vi "4.0.3_Airwatts_Finetune.vi"(6 "Data in":T1, 8 "error in (no error)":errorcluster, 9 "AllControls In":T2, 10 "?":T3, 11 "Message Queue out":T4) -> (0 "error out":errorcluster, 1 "Flow":string, 2 "Data":T3, 3 "Message Queue Out":T4, 4 "Data out":T1)   [LabVIEW 2017]
uses:
  Depends/AMC/subVIs/TypeDefs/amc_Message Queue.ctl
  Depends/AMC/subVIs/TypeDefs/amc_Message.ctl
  Depends/Tools/Keyed Array/Tools_KeyedArray KeyedArray.ctl
  Ctrls/Data.ctl
  Ctrls/AllControls.ctl
  Ctrls/CSV_Data.ctl
  DIPC 692 Daemon API/typdef/get_parameter.ctl
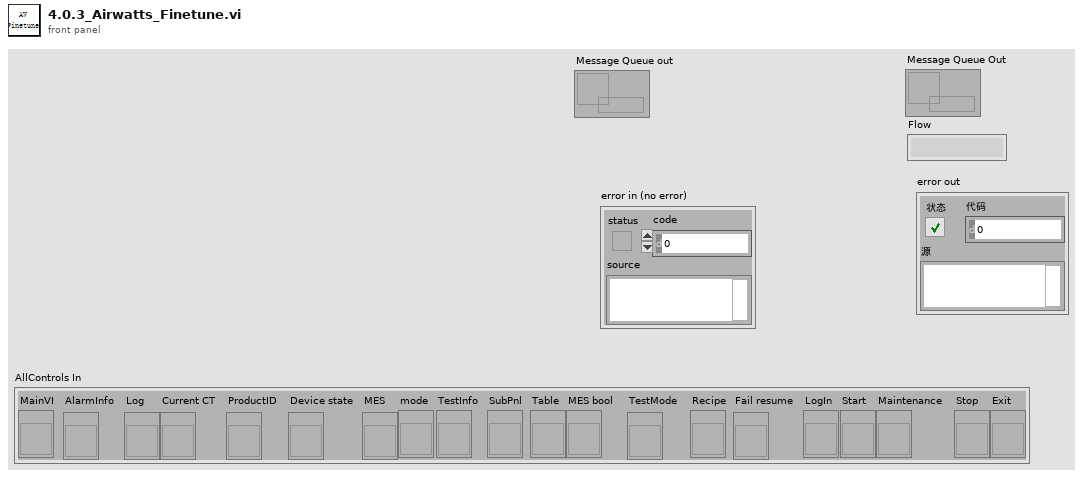
[diagram p1: front panel]
types:
  T1 = typedef "CSV_Data.ctl" = cluster{"Initialisation":cluster{"LMT - Connect UUT (con COM)":string, "LMT - Software Version (rrel)":string, "LMT - Write SKU file (wskuc)":string, "LMT - SKU file name":string, "Connect UUT DDM":string, "Read DDM EOL Timestamp - Mode":string, "Read DDM EOL Timestamp - Timestamp":string, "Read DDM EOL Timestamp - Rig ID":string, "Read DDM EOL Timestamp - Passmark ID":string, "Read DDM EOL Timestamp - Passmark Rev":string, "Software Version before flashing":string, "Read Hardware Serial":string, "UUT DDM SN":string, "Compare DDM SN with MES SN":string, "Backup PCBA Calibration EEPROM Response - CAL":string, "Flash Firmware Version":string, "Check SW Version":string, "Read DDM SW Version after flashing":string, "Set SKU Config":string, "Ready Status":string, "Set Device Mode to EOL":string, "DDM Parameter - Voltage":string, "DDM Parameter - Current":string, "DDM Parameter - Power":string, "DDM Parameter - Speed":string, "DDM Parameter - Pressure":string, "Tester Parameter - Voltage":string, "Tester Parameter - Current":string, "Tester Parameter - Power":string, "Tester Parameter - Ambient Pressure":string, "Tester Parameter - Ambient Temperature":string, "Calculated Parameter - DDM Pressure Corrected":string, "Calculated Parameter - DDM Real Power":string, "Calculated Parameter - Delta V":string}, "BEMF_Calibration":cluster{"Calibration Result - eol_cold_bemf_temp":string, "DDM Ambient Temp":string, "Restriction Plate Diameter":string, "Calibration Result - eol_bemf_mp_cold_coef_a":string, "Calibration Result - eol_bemf_mp_cold_coef_b":string, "Calibration Result - eol_bemf_mp_cold_coef_c":string, "Calibration Result - eol_bemf_lsi_cold_ref_coeffs":string, "Get - Calibration Result - eol_bemf_lsi_speed":string, "Get - Calibration Result - eol_bemf_lsi_integral_0":string, "Calibration Result - eol_bemf_lsi_integral_1":string, "Get - Calibration Result - eol_bemf_lsi_integral_2":string, "Get - Calibration Result - eol_cold_bemf":string, "Get - Calibration Result - eol_cold_bemf_fisf":string, "Finalise Calibration":string, "Compare -Calibration Result - eol_cold_bemf":string, "Compare -Calibration Result - eol_cold_bemf_fisf":string}, "ECO":cluster{"Reset Power Tune":string, "Reset BEMF FISF Calibration":string, "Restriction Plate Diameter":string, "ECO - Stabilisation Time":string, "ECO - DDM Parameter - Voltage":string, "ECO - DDM Parameter - Current":string, "ECO - DDM Parameter - Power":string, "ECO - DDM Parameter - Measured Power":string, "ECO - DDM Parameter - Speed":string, "ECO - DDM Parameter - Pressure":string, "ECO - Tester Parameter - Voltage":string, "ECO - Tester Parameter - Current":string, "ECO - Tester Parameter - Power":string, "ECO - Tester Parameter - Ambient Pressure":string, "ECO - Tester Parameter - Ambient Temperature":string, "ECO - Tester Parameter - Ambient Humidity":string, "ECO - Calculated Parameter - DDM Pressure Corrected":string, "ECO - Calculated Parameter - DDM Real Power":string, "ECO - Calculated Parameter - Delta V":string, "ECO - Calculated Parameter - Flowrate":string, "ECO - Calculated Parameter - Airwatt":string, "ECO - Formula":string, "PT ECO - Power Tune Mode Status":string}, "BOOST":cluster{"Restriction Plate Diameter":string, "BOOST - Stabilisation Time":string, "BOOST - DDM Parameter - Voltage":string, "BOOST - DDM Parameter - Current":string, "BOOST - DDM Parameter - Power":string, "BOOST - DDM Parameter - Measured Power":string, "BOOST - DDM Parameter - Speed":string, "BOOST - DDM Parameter - Pressure":string, "BOOST - Tester Parameter - Voltage":string, "BOOST - Tester Parameter - Current":string, "BOOST - Tester Parameter - Power":string, "BOOST - Tester Parameter - Ambient Pressure":string, "BOOST - Tester Parameter - Ambient Temperature":string, "BOOST - Tester Parameter - Ambient Humidity":string, "BOOST - Calculated Parameter - DDM Pressure Corrected":string, "BOOST - Calculated Parameter - DDM Real Power":string, "BOOST - Calculated Parameter - Delta V":string, "BOOST - Calculated Parameter - Flowrate":string, "BOOST - Calculated Parameter - Airwatt":string, "BOOST - Get AM Presence":string, "Air Muscle Turn Off Status":string, "BOOST - Air Muscle Calculated Parameter - Airwatt B":string, "BOOST - Air Muscle Calculate Airwatt Delta":string, "PT BOOST - Power Tune Mode Status":string, "Finalise Calibration":string, "ECO - Get AW Calibration value":string, "BOOST - Get AW Calibration value":string}, "MAX":cluster{"Restriction Plate Diameter":string, "MAX - Stabilisation Time":string, "Get Average Delta Tmag (LSIdelta_FISFdelta_LSItmag_FISFtmag_IIRtmag)":string, "Get Average Delta Tmag FISF":string, "MAX - DDM Parameter - Voltage":string, "MAX - DDM Parameter - Current":string, "MAX - DDM Parameter - Power":string, "MAX - DDM Parameter - Measured Power":string, "MAX - DDM Parameter - Speed":string, "MAX - DDM Parameter - Pressure":string, "MAX - Tester Parameter - Voltage":string, "MAX - Tester Parameter - Current":string, "MAX - Tester Parameter - Power":string, "MAX - Tester Parameter - Ambient Pressure":string, "MAX - Tester Parameter - Ambient Temperature":string, "MAX - Tester Parameter - Ambient Humidity":string, "MAX - Calculated Parameter - DDM Pressure Corrected":string, "MAX - Calculated Parameter - DDM Real Power":string, "MAX - Calculated Parameter - Delta V":string, "MAX - Calculated Parameter - Flowrate":string, "MAX - Calculated Parameter - Airwatt":string, "MAX_FISF_Check_Average_Delta_Tmag":string, "MAX - FISF - BEMF Finetune Result":string, "MAX tune - Delta P1":string, "MAX tune - Calculated Parameter - Airwatt":string, "Calculate Delta Airwatts - MAX finetune - Delta P2":string, "MAX finetune - DDM Parameter - Voltage":string, "MAX finetune - DDM Parameter - Current":string, "MAX finetune - DDM Parameter - Power":string, "MAX finetune - DDM Parameter - Measured Power":string, "MAX finetune - DDM Parameter - Speed":string, "MAX finetune - DDM Parameter - Pressure":string, "MAX finetune - Tester Parameter - Voltage":string, "MAX finetune - Tester Parameter - Current":string, "MAX finetune - Tester Parameter - Power":string, "MAX finetune - Tester Parameter - Ambient Pressure":string, "MAX finetune - Tester Parameter - Ambient Temperature":string, "MAX finetune - Tester Parameter - Ambient Humidity":string, "MAX finetune - Calculated Parameter - DDM Pressure Corrected":string, "MAX finetune - Calculated Parameter - DDM Real Power":string, "MAX finetune - Calculated Parameter - Delta V":string, "MAX finetune - Calculated Parameter - Flowrate":string, "MAX finetune - Calculated Parameter - Airwatt":string, "Check Derate Result":string, "Delta Tmag FISF":string, "Get Hot BEMF Result":string, "Calculate delta Pressure":string, "Finalise Calibration":string, "Calculate & Check Delta BEMF":string, "Delta P Airwatts Value":string}, "LL":cluster{"DDM Ambient Temp":string, "Restriction Plate Diameter":string, "LL - DDM Parameter - Voltage":string, "LL - DDM Parameter - Current":string, "LL - DDM Parameter - Power":string, "LL - DDM Parameter - Measured Power":string, "LL - DDM Parameter - Speed":string, "LL - DDM Parameter - Pressure":string, "LL - Tester Parameter - Voltage":string, "LL - Tester Parameter - Current":string, "LL - Tester Parameter - Power":string, "LL - DDM Real Power":string, "LL - Calibrate Task Detect LL":string}, "HL":cluster{"HL - DDM Parameter - Voltage":string, "HL - DDM Parameter - Current":string, "HL - DDM Parameter - Power":string, "HL - DDM Parameter - Measured Power":string, "HL - DDM Parameter - Speed":string, "HL - DDM Parameter - Pressure":string, "HL - Tester Parameter - Voltage":string, "HL - Tester Parameter - Current":string, "HL - Tester Parameter - Power":string, "HL - DDM Real Power":string, "HL - Calibrate Task Detect HL":string}, "LH":cluster{"Restriction Plate Diameter":string, "LH - DDM Parameter - Voltage":string, "LH - DDM Parameter - Current":string, "LH - DDM Parameter - Power":string, "LH - DDM Parameter - Measured Power":string, "LH - DDM Parameter - Speed":string, "LH - DDM Parameter - Pressure":string, "LH - Tester Parameter - Voltage":string, "LH - Tester Parameter - Current":string, "LH - Tester Parameter - Power":string, "LH - DDM Real Power":string, "LH - Calibrate Task Detect LH":string}, "HH":cluster{"HH - DDM Parameter - Voltage":string, "HH - DDM Parameter - Current":string, "HH - DDM Parameter - Power":string, "HH - DDM Parameter - Measured Power":string, "HH - DDM Parameter - Speed":string, "HH - DDM Parameter - Pressure":string, "HH - Tester Parameter - Voltage":string, "HH - Tester Parameter - Current":string, "HH - Tester Parameter - Power":string, "HH - DDM Real Power":string, "HH - Calibrate Task Detect HH":string}, "Inlet Blockage Calibration":cluster{"Inlet Blockage Calibration - DDM Parameter - Voltage":string, "Inlet Blockage Calibration - DDM Parameter - Current":string, "Inlet Blockage Calibration - DDM Parameter - Power":string, "Inlet Blockage Calibration - DDM Parameter - Measured Power":string, "Inlet Blockage Calibration - DDM Parameter - Speed":string, "Inlet Blockage Calibration - DDM Parameter - Pressure":string, "Inlet Blockage Calibration - Tester Parameter - Voltage":string, "Inlet Blockage Calibration - Tester Parameter - Current":string, "Inlet Blockage Calibration - Tester Parameter - Power":string, "Inlet Blockage Calibration - DDM Real Power":string, "Calibration Inlet Blockage_E":string, "Finalise Calibration":string, "Get Task Detect LL":string, "Get Task Detect HL":string, "Get Task Detect LH":string, "Get Task Detect HH":string, "Calibration Inlet Blockage":string, "Calibration eol cold bemf temp":string}, "GOOD":cluster{"GOOD UNIT - Clear EEPROM Error Log":string, "GOOD UNIT - Write Product Timestamp - Mode":string, "GOOD UNIT - Write Product Timestamp - Timestamp":string, "GOOD UNIT - Write Product Timestamp - Rig ID":string, "GOOD UNIT - Write Product Timestamp - Passmark ID":string, "GOOD UNIT - Write Product Timestamp - Passmark Rev":string, "GOOD UNIT - Set Device Mode to PROD":string, "GOOD UNIT - Backup PCBA Calibration EEPROM Response":string, "GOOD UNIT - Check Security Bit":string, "GOOD UNIT - Set Calibration Lock":string, "GOOD UNIT - Get_Calibration_Lock":string, "GOOD UNIT - Disconnect UUT":string}, "NG":cluster{"NG UNIT - Read NVM Error":string, "NG UNIT - Set Device Mode to FCT":string, "NG UNIT - Backup PCBA Calibration EEPROM Response - CAL":string, "NG UNIT - Backup PCBA Calibration EEPROM Response - ERROR":string, "NG UNIT - Backup PCBA Calibration EEPROM Response - USAGE":string, "NG UNIT - Disconnect UUT":string}, "SN":string, "Table":string[][], "Count":cluster{"Total":i32, "OK":i32, "NG":i32, "Yield":dbl}, "Start Time":timestamp, "daemon reference":refnum<k5>, "CT":dbl, "Config":string[][], "OK/NG":bool, "Station ID":string, "MES DDM SN":string, "MES PCBA SN":string, "Retest":string, "UID":string, "Initialisation_Status":cluster{"LMT - Connect UUT (con COM)":string, "LMT - Software Version (rrel)":string, "LMT - Write SKU file (wskuc)":string, "LMT - SKU file name":string, "Connect UUT DDM":string, "Read DDM EOL Timestamp - Mode":string, "Read DDM EOL Timestamp - Timestamp":string, "Read DDM EOL Timestamp - Rig ID":string, "Read DDM EOL Timestamp - Passmark ID":string, "Read DDM EOL Timestamp - Passmark Rev":string, "Software Version before flashing":string, "Read Hardware Serial":string, "UUT DDM SN":string, "Compare DDM SN with MES SN":string, "Backup PCBA Calibration EEPROM Response - CAL":string, "Flash Firmware Version":string, "Check SW Version":string, "Read DDM SW Version after flashing":string, "Set SKU Config":string, "Ready Status":string, "Set Device Mode to EOL":string, "DDM Parameter - Voltage":string, "DDM Parameter - Current":string, "DDM Parameter - Power":string, "DDM Parameter - Speed":string, "DDM Parameter - Pressure":string, "Tester Parameter - Voltage":string, "Tester Parameter - Current":string, "Tester Parameter - Power":string, "Tester Parameter - Ambient Pressure":string, "Tester Parameter - Ambient Temperature":string, "Calculated Parameter - DDM Pressure Corrected":string, "Calculated Parameter - DDM Real Power":string, "Calculated Parameter - Delta V":string}, "BEMF_Calibration_Status":cluster{"Calibration Result - eol_cold_bemf_temp":string, "DDM Ambient Temp":string, "Restriction Plate Diameter":string, "Calibration Result - eol_bemf_mp_cold_coef_a":string, "Calibration Result - eol_bemf_mp_cold_coef_b":string, "Calibration Result - eol_bemf_mp_cold_coef_c":string, "Calibration Result - eol_bemf_lsi_cold_ref_coeffs":string, "Get - Calibration Result - eol_bemf_lsi_speed":string, "Get - Calibration Result - eol_bemf_lsi_integral_0":string, "Calibration Result - eol_bemf_lsi_integral_1":string, "Get - Calibration Result - eol_bemf_lsi_integral_2":string, "Get - Calibration Result - eol_cold_bemf":string, "Get - Calibration Result - eol_cold_bemf_fisf":string, "Finalise Calibration":string, "Compare -Calibration Result - eol_cold_bemf":string, "Compare -Calibration Result - eol_cold_bemf_fisf":string}, "ECO_Status":cluster{"Reset Power Tune":string, "Reset BEMF FISF Calibration":string, "Restriction Plate Diameter":string, "ECO - Stabilisation Time":string, "ECO - DDM Parameter - Voltage":string, "ECO - DDM Parameter - Current":string, "ECO - DDM Parameter - Power":string, "ECO - DDM Parameter - Measured Power":string, "ECO - DDM Parameter - Speed":string, "ECO - DDM Parameter - Pressure":string, "ECO - Tester Parameter - Voltage":string, "ECO - Tester Parameter - Current":string, "ECO - Tester Parameter - Power":string, "ECO - Tester Parameter - Ambient Pressure":string, "ECO - Tester Parameter - Ambient Temperature":string, "ECO - Tester Parameter - Ambient Humidity":string, "ECO - Calculated Parameter - DDM Pressure Corrected":string, "ECO - Calculated Parameter - DDM Real Power":string, "ECO - Calculated Parameter - Delta V":string, "ECO - Calculated Parameter - Flowrate":string, "ECO - Calculated Parameter - Airwatt":string, "ECO - Formula":string, "PT ECO - Power Tune Mode Status":string}, "BOOST_Status":cluster{"Restriction Plate Diameter":string, "BOOST - Stabilisation Time":string, "BOOST - DDM Parameter - Voltage":string, "BOOST - DDM Parameter - Current":string, "BOOST - DDM Parameter - Power":string, "BOOST - DDM Parameter - Measured Power":string, "BOOST - DDM Parameter - Speed":string, "BOOST - DDM Parameter - Pressure":string, "BOOST - Tester Parameter - Voltage":string, "BOOST - Tester Parameter - Current":string, "BOOST - Tester Parameter - Power":string, "BOOST - Tester Parameter - Ambient Pressure":string, "BOOST - Tester Parameter - Ambient Temperature":string, "BOOST - Tester Parameter - Ambient Humidity":string, "BOOST - Calculated Parameter - DDM Pressure Corrected":string, "BOOST - Calculated Parameter - DDM Real Power":string, "BOOST - Calculated Parameter - Delta V":string, "BOOST - Calculated Parameter - Flowrate":string, "BOOST - Calculated Parameter - Airwatt":string, "BOOST - Get AM Presence":string, "Air Muscle Turn Off Status":string, "BOOST - Air Muscle Calculated Parameter - Airwatt B":string, "BOOST - Air Muscle Calculate Airwatt Delta":string, "PT BOOST - Power Tune Mode Status":string, "Finalise Calibration":string, "ECO - Get AW Calibration value":string, "BOOST - Get AW Calibration value":string}, "MAX_Status":cluster{"Restriction Plate Diameter":string, "MAX - Stabilisation Time":string, "Get Average Delta Tmag (LSIdelta_FISFdelta_LSItmag_FISFtmag_IIRtmag)":string, "Get Average Delta Tmag FISF":string, "MAX - DDM Parameter - Voltage":string, "MAX - DDM Parameter - Current":string, "MAX - DDM Parameter - Power":string, "MAX - DDM Parameter - Measured Power":string, "MAX - DDM Parameter - Speed":string, "MAX - DDM Parameter - Pressure":string, "MAX - Tester Parameter - Voltage":string, "MAX - Tester Parameter - Current":string, "MAX - Tester Parameter - Power":string, "MAX - Tester Parameter - Ambient Pressure":string, "MAX - Tester Parameter - Ambient Temperature":string, "MAX - Tester Parameter - Ambient Humidity":string, "MAX - Calculated Parameter - DDM Pressure Corrected":string, "MAX - Calculated Parameter - DDM Real Power":string, "MAX - Calculated Parameter - Delta V":string, "MAX - Calculated Parameter - Flowrate":string, "MAX - Calculated Parameter - Airwatt":string, "MAX_FISF_Check_Average_Delta_Tmag":string, "MAX - FISF - BEMF Finetune Result":string, "MAX tune - Delta P1":string, "MAX tune - Calculated Parameter - Airwatt":string, "Calculate Delta Airwatts - MAX finetune - Delta P2":string, "MAX finetune - DDM Parameter - Voltage":string, "MAX finetune - DDM Parameter - Current":string, "MAX finetune - DDM Parameter - Power":string, "MAX finetune - DDM Parameter - Measured Power":string, "MAX finetune - DDM Parameter - Speed":string, "MAX finetune - DDM Parameter - Pressure":string, "MAX finetune - Tester Parameter - Voltage":string, "MAX finetune - Tester Parameter - Current":string, "MAX finetune - Tester Parameter - Power":string, "MAX finetune - Tester Parameter - Ambient Pressure":string, "MAX finetune - Tester Parameter - Ambient Temperature":string, "MAX finetune - Tester Parameter - Ambient Humidity":string, "MAX finetune - Calculated Parameter - DDM Pressure Corrected":string, "MAX finetune - Calculated Parameter - DDM Real Power":string, "MAX finetune - Calculated Parameter - Delta V":string, "MAX finetune - Calculated Parameter - Flowrate":string, "MAX finetune - Calculated Parameter - Airwatt":string, "Check Derate Result":string, "Delta Tmag FISF":string, "Get Hot BEMF Result":string, "Calculate delta Pressure":string, "Finalise Calibration":string, "Calculate & Check Delta BEMF":string, "Delta P Airwatts Value":string}, "LL_Status":cluster{"DDM Ambient Temp":string, "Restriction Plate Diameter":string, "LL - DDM Parameter - Voltage":string, "LL - DDM Parameter - Current":string, "LL - DDM Parameter - Power":string, "LL - DDM Parameter - Measured Power":string, "LL - DDM Parameter - Speed":string, "LL - DDM Parameter - Pressure":string, "LL - Tester Parameter - Voltage":string, "LL - Tester Parameter - Current":string, "LL - Tester Parameter - Power":string, "LL - DDM Real Power":string, "LL - Calibrate Task Detect LL":string}, "HL_Status":cluster{"HL - DDM Parameter - Voltage":string, "HL - DDM Parameter - Current":string, "HL - DDM Parameter - Power":string, "HL - DDM Parameter - Measured Power":string, "HL - DDM Parameter - Speed":string, "HL - DDM Parameter - Pressure":string, "HL - Tester Parameter - Voltage":string, "HL - Tester Parameter - Current":string, "HL - Tester Parameter - Power":string, "HL - DDM Real Power":string, "HL - Calibrate Task Detect HL":string}, "LH_Status":cluster{"Restriction Plate Diameter":string, "LH - DDM Parameter - Voltage":string, "LH - DDM Parameter - Current":string, "LH - DDM Parameter - Power":string, "LH - DDM Parameter - Measured Power":string, "LH - DDM Parameter - Speed":string, "LH - DDM Parameter - Pressure":string, "LH - Tester Parameter - Voltage":string, "LH - Tester Parameter - Current":string, "LH - Tester Parameter - Power":string, "LH - DDM Real Power":string, "LH - Calibrate Task Detect LH":string}, "HH_Status":cluster{"HH - DDM Parameter - Voltage":string, "HH - DDM Parameter - Current":string, "HH - DDM Parameter - Power":string, "HH - DDM Parameter - Measured Power":string, "HH - DDM Parameter - Speed":string, "HH - DDM Parameter - Pressure":string, "HH - Tester Parameter - Voltage":string, "HH - Tester Parameter - Current":string, "HH - Tester Parameter - Power":string, "HH - DDM Real Power":string, "HH - Calibrate Task Detect HH":string}, "Inlet Blockage Calibration_Status":cluster{"Inlet Blockage Calibration - DDM Parameter - Voltage":string, "Inlet Blockage Calibration - DDM Parameter - Current":string, "Inlet Blockage Calibration - DDM Parameter - Power":string, "Inlet Blockage Calibration - DDM Parameter - Measured Power":string, "Inlet Blockage Calibration - DDM Parameter - Speed":string, "Inlet Blockage Calibration - DDM Parameter - Pressure":string, "Inlet Blockage Calibration - Tester Parameter - Voltage":string, "Inlet Blockage Calibration - Tester Parameter - Current":string, "Inlet Blockage Calibration - Tester Parameter - Power":string, "Inlet Blockage Calibration - DDM Real Power":string, "Calibration Inlet Blockage_E":string, "Finalise Calibration":string, "Get Task Detect LL":string, "Get Task Detect HL":string, "Get Task Detect LH":string, "Get Task Detect HH":string, "Calibration Inlet Blockage":string, "Calibration eol cold bemf temp":string}, "GOOD_Status":cluster{"GOOD UNIT - Clear EEPROM Error Log":string, "GOOD UNIT - Write Product Timestamp - Mode":string, "GOOD UNIT - Write Product Timestamp - Timestamp":string, "GOOD UNIT - Write Product Timestamp - Rig ID":string, "GOOD UNIT - Write Product Timestamp - Passmark ID":string, "GOOD UNIT - Write Product Timestamp - Passmark Rev":string, "GOOD UNIT - Set Device Mode to PROD":string, "GOOD UNIT - Backup PCBA Calibration EEPROM Response":string, "GOOD UNIT - Check Security Bit":string, "GOOD UNIT - Set Calibration Lock":string, "GOOD UNIT - Get_Calibration_Lock":string, "GOOD UNIT - Disconnect UUT":string}, "NG_Status":cluster{"NG UNIT - Read NVM Error":string, "NG UNIT - Set Device Mode to FCT":string, "NG UNIT - Backup PCBA Calibration EEPROM Response - CAL":string, "NG UNIT - Backup PCBA Calibration EEPROM Response - ERROR":string, "NG UNIT - Backup PCBA Calibration EEPROM Response - USAGE":string, "NG UNIT - Disconnect UUT":string}, "SKU":string, "Plate_Diameter":string, "Alarm":string}
  T2 = typedef "AllControls.ctl" = cluster{"MainVI":refnum<vi>, "AlarmInfo":refnum<vi>, "Log":refnum<vi>, "Current CT":refnum<vi>, "ProductID":refnum<vi>, "Device state":refnum<vi>, "MES":refnum<vi>, "mode":refnum<vi>, "TestInfo":refnum<vi>, "SubPnl":refnum<vi>, "Table":refnum<vi>, "MES bool":refnum<vi>, "TestMode":refnum<vi>, "Recipe":refnum<vi>, "Fail resume":refnum<vi>, "LogIn":refnum<vi>, "Start":refnum<vi>, "Maintenance":refnum<vi>, "Stop":refnum<vi>, "Exit":refnum<vi>}
  T3 = typedef "Data.ctl" = cluster{"Initialisation":cluster{"DDM_Parameter":dbl[], "DDM_Parameter_status":bool[], "Get_Tester_Parameter":dbl[], "Get_Tester_Parameter_status":bool[], "Cal_Tester_Parameter":dbl[], "Cal_Tester_Parameter_status":bool[], "sw_version_before_status":bool, "sw_version_after_status":bool, "Set_SKU_Config_With_LMT_status":bool, "FCT_timestamp_status":bool, "LMT_Connect_to_UUT_status":bool}, "BEMF_Calibration":cluster{"Read_ambient_temperature":dbl, "Calibration_Vaule":dbl[], "Calibration_Vaule _B":dbl[], "Calibration_Vaule_status":bool[], "Calibration_Vaule_B_status":bool[]}, "ECO":cluster{"DDM_Parameter":dbl[], "DDM_Parameter_status":bool[], "Get_Tester_Parameter":dbl[], "Get_Tester_Parameter_status":bool[], "Cal_Tester_Parameter":dbl[], "Cal_Tester_Parameter_status":bool[], "DDM_Parameter_after_power_tune":dbl[], "Get_Tester_Parameter_after_power_tune":dbl[], "Cal_Tester_Parameter_after_power_tune":dbl[], "Cal_Tester_Parameter_after_power_tune_status":bool[], "Delta_P":dbl}, "BOOST":cluster{"DDM_Parameter":dbl[], "DDM_Parameter_status":bool[], "Get_Tester_Parameter":dbl[], "Get_Tester_Parameter_status":bool[], "Cal_Tester_Parameter":dbl[], "Cal_Tester_Parameter_status":bool[], "DDM_Parameter_after_power_tune":dbl[], "Get_Tester_Parameter_after_power_tune":dbl[], "Cal_Tester_Parameter_after_power_tune":dbl[], "Cal_Tester_Parameter_after_power_tune_status":bool[], "airwatts_am_off":dbl, "AW_Delta_(AM_on_and_off)":dbl, "AW_Delta_(AM_on_and_off)_Status":bool, "Delta_P":dbl}, "MAX":cluster{"Average_Tmag_Data":cluster{"LSI Delta in degC":dbl, "FISF Delta in degc":dbl, "LSI Tmag in degC":dbl, "Fisf Tmag in degC":dbl, "IIR Tmag in degC":dbl}, "DDM_Parameter":dbl[], "DDM_Parameter_status":bool[], "Get_Tester_Parameter":dbl[], "Get_Tester_Parameter_status":bool[], "Cal_Tester_Parameter":dbl[], "BEMF_Finetune":cluster{"eol_bemf_mp_cold_coef_c":dbl, "eol_cold_bemf_fisf_offset":dbl}, "AW_Tune":cluster{"delta_P1":dbl, "delta_P_Setting":dbl}, "DDM_Parameter_after_Airwatts_Tune":dbl[], "Get_Tester_Parameter_after_Airwatts_Tune":dbl[], "Cal_Tester_Parameter_after_Airwatts_Tune":dbl[], "DDM_Parameter_after_Airwatts_Finetune":dbl[], "Get_Tester_Parameter_after_Airwatts_Finetune":dbl[], "Cal_Tester_Parameter_after_Airwatts_Finetune":dbl[], "AW_Finetune":cluster{"delta_P2":dbl, "delta_P_Setting":dbl}, "Delta_Tmag_after_tune":cluster{"LSI Delta in degC":dbl, "FISF Delta in degc":dbl, "LSI Tmag in degC":dbl, "Fisf Tmag in degC":dbl, "IIR Tmag in degC":dbl}, "Hot Bemf in mV":dbl, "DDM_Pressure":dbl, "Delta_Pressure":dbl, " Cold Bemf in mV":dbl, " delta Bemf":dbl, " delta p":dbl, "Delta_Pressure_status":bool, " delta Bemf_status":bool, "LSI Delta in degC_status":bool, "FISF Delta in degc_status":bool, "Max_check_derate_status_status":bool, "Average_All_data":dbl[][], "Average_Tmag_Data_status":bool[], "Average_Tmag_Data_after_tune_status":bool[], "Cal_Tester_Parameter_status":bool[], "Cal_Tester_Parameter_status_after_Airwatts_Tune":bool[], "Cal_Tester_Parameter_status_after_Airwatts_FineTune":bool[]}, "Task_Detect_Calib":cluster{"LL":cluster{"DDM_Parameter":dbl[], "DDM_Parameter_status":bool[], "Get_Tester_Parameter":dbl[], "Get_Tester_Parameter_status":bool[], "Set_task_detect_A":dbl, "Set_task_detect_A_Status":bool}, "HL":cluster{"DDM_Parameter":dbl[], "DDM_Parameter_status":bool[], "Get_Tester_Parameter":dbl[], "Get_Tester_Parameter_status":bool[], "Set_task_detect_B":dbl, "Set_task_detect_B_Status":bool}, "LH":cluster{"DDM_Parameter":dbl[], "DDM_Parameter_status":bool[], "Get_Tester_Parameter":dbl[], "Get_Tester_Parameter_status":bool[], "Set_task_detect_C":dbl, "Set_task_detect_C_Status":bool}, "HH":cluster{"DDM_Parameter":dbl[], "DDM_Parameter_status":bool[], "Get_Tester_Parameter":dbl[], "Get_Tester_Parameter_status":bool[], "Set_task_detect_D":dbl, "Read_and_check_calibration_Status":bool[], "Set_task_detect_D_Status":bool}, "Get_eol_inlet_blockage_E":dbl, "Calib_vaule":cluster{"Get_task_detect_LL":dbl, "Get_task_detect_HL":dbl, "Get_task_detect_LH":dbl, "Get_task_detect_HH":dbl, "eol_inlet_blockage":dbl, "eol_code_bemf_temp":dbl}, "calibrated temp":dbl, "Inlet_Blockage_Calibration":cluster{"DDM_Parameter":dbl[], "DDM_Parameter_status":bool[], "Get_Tester_Parameter":dbl[], "Get_Tester_Parameter_status":bool[]}, "Get_eol_inlet_blockage_E_Status":bool}, "good":cluster{"Write_Product_TS":cluster{"TIMESTAMP":i64, "RIG_ID":i64, "PASSMARK_ID":i64, "PASSMARK_REV":i64}, "Read_Product_TS":cluster{"TIMESTAMP":i64, "RIG_ID":i64, "PASSMARK_ID":i64, "PASSMARK_REV":i64}, "Good_Check_Secuity_Bit_Stauts":bool}}
  T4 = typedef "amc_Message Queue.ctl" = refnum<queue>
  T5 = typedef "HD Config.ctl" = cluster{" PC":cluster{"PC Address":u8[], "PC Port":i32}, "FCO":cluster{"COM":refnum<visa-resource-name>, "Baudrate":u32}, "DC Power ":cluster{"COM":refnum<visa-resource-name>, "Baudrate":u32}, "PW3336":cluster{"COM":refnum<visa-resource-name>, "Baudrate":u32}, "Lefoo":cluster{"COM":refnum<visa-resource-name>, "Baudrate":u32}, "AI Model":cluster{"COM":refnum<visa-resource-name>, "Baudrate":u32}, "DIPC":cluster{"COM":refnum<visa-resource-name>}, "RFID":cluster{"IP Address":string, "Port":u16, "Retry":u16}, "Motor":cluster{"COM":refnum<visa-resource-name>, "Baudrate":u32}, "Fail_resume_mode":bool, "GRR":bool}
  T6 = cluster{"real_ddm_power_a_in_W":dbl, "real_ddm_power_b_in_W":dbl, "Target_AW":dbl, "AW extra":dbl, "latest_AW":dbl, "Correction_Factor":dbl, "P_extra in W":dbl, "delta_P index":dbl}
  T7 = typedef "get_parameter.ctl" = string
  T8 = cluster{"real_ddm_power_a_in_W":string, "real_ddm_power_b_in_W":string, "Target_AW":string, "AW extra":string, "latest_AW":string, "Correction_Factor":string, "P_extra in W":string, "delta_P index":string}
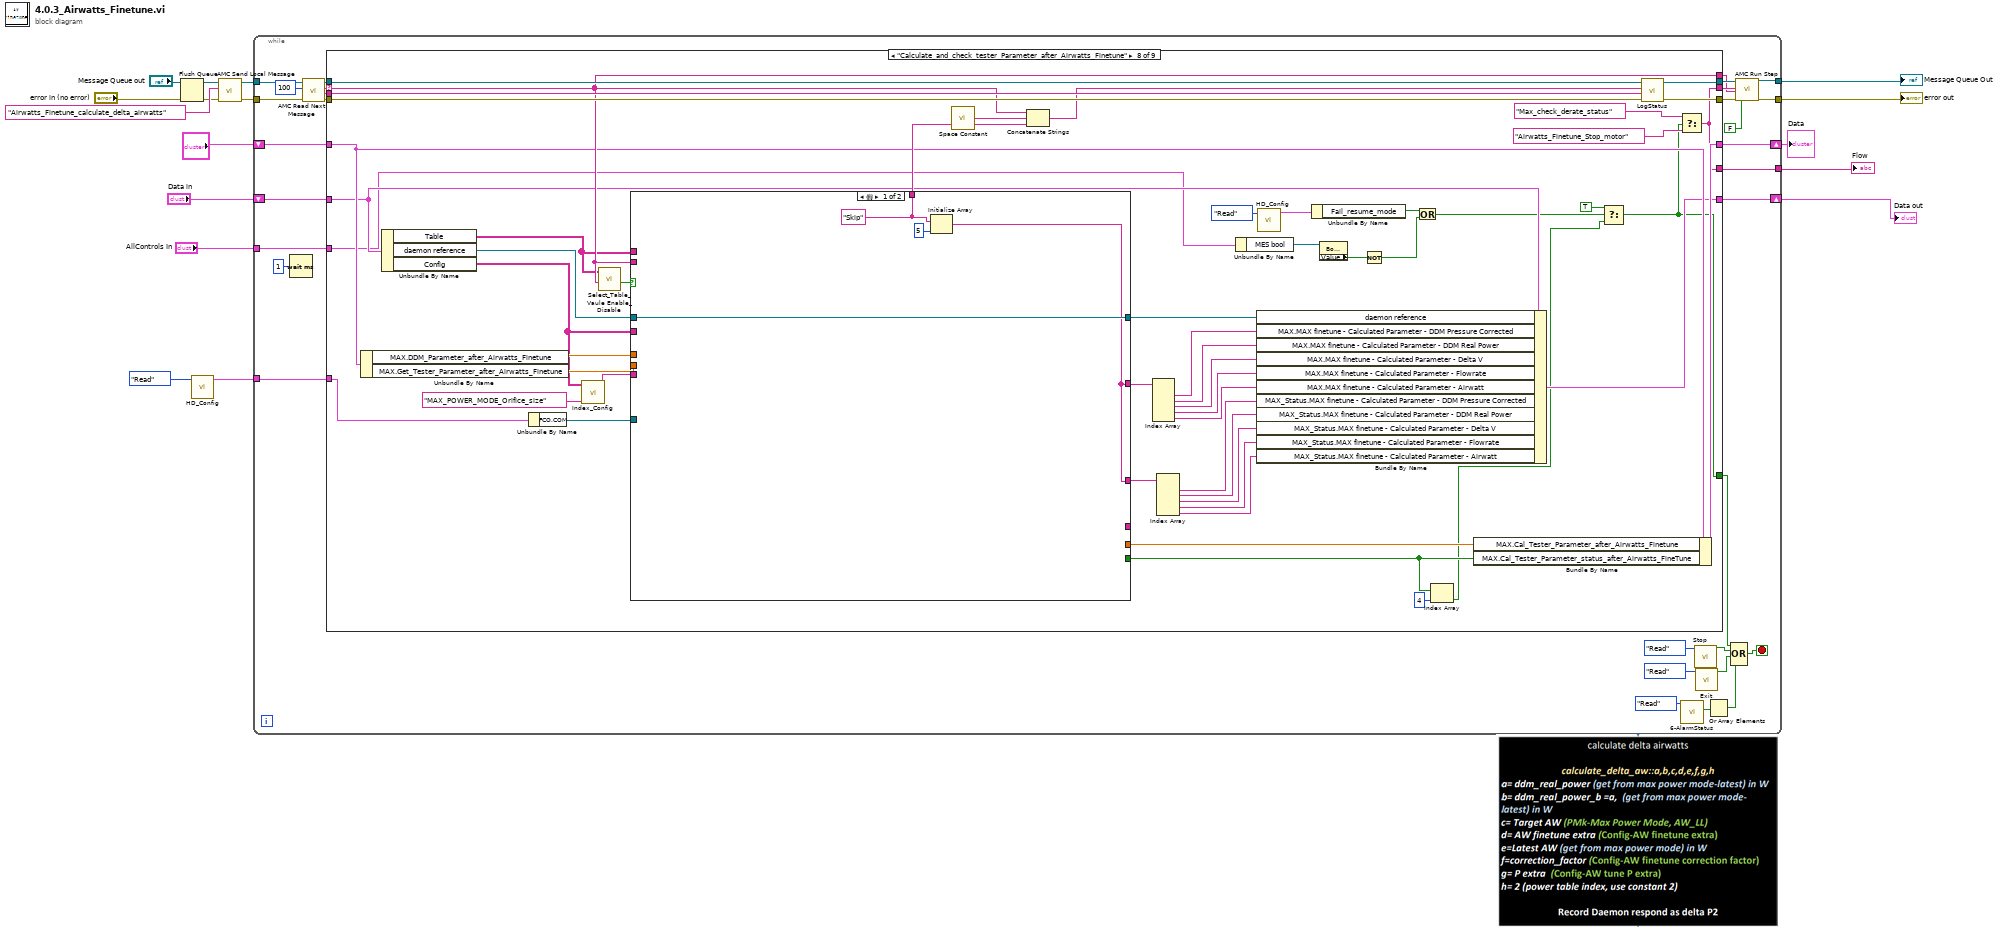
[diagram p0: block diagram]
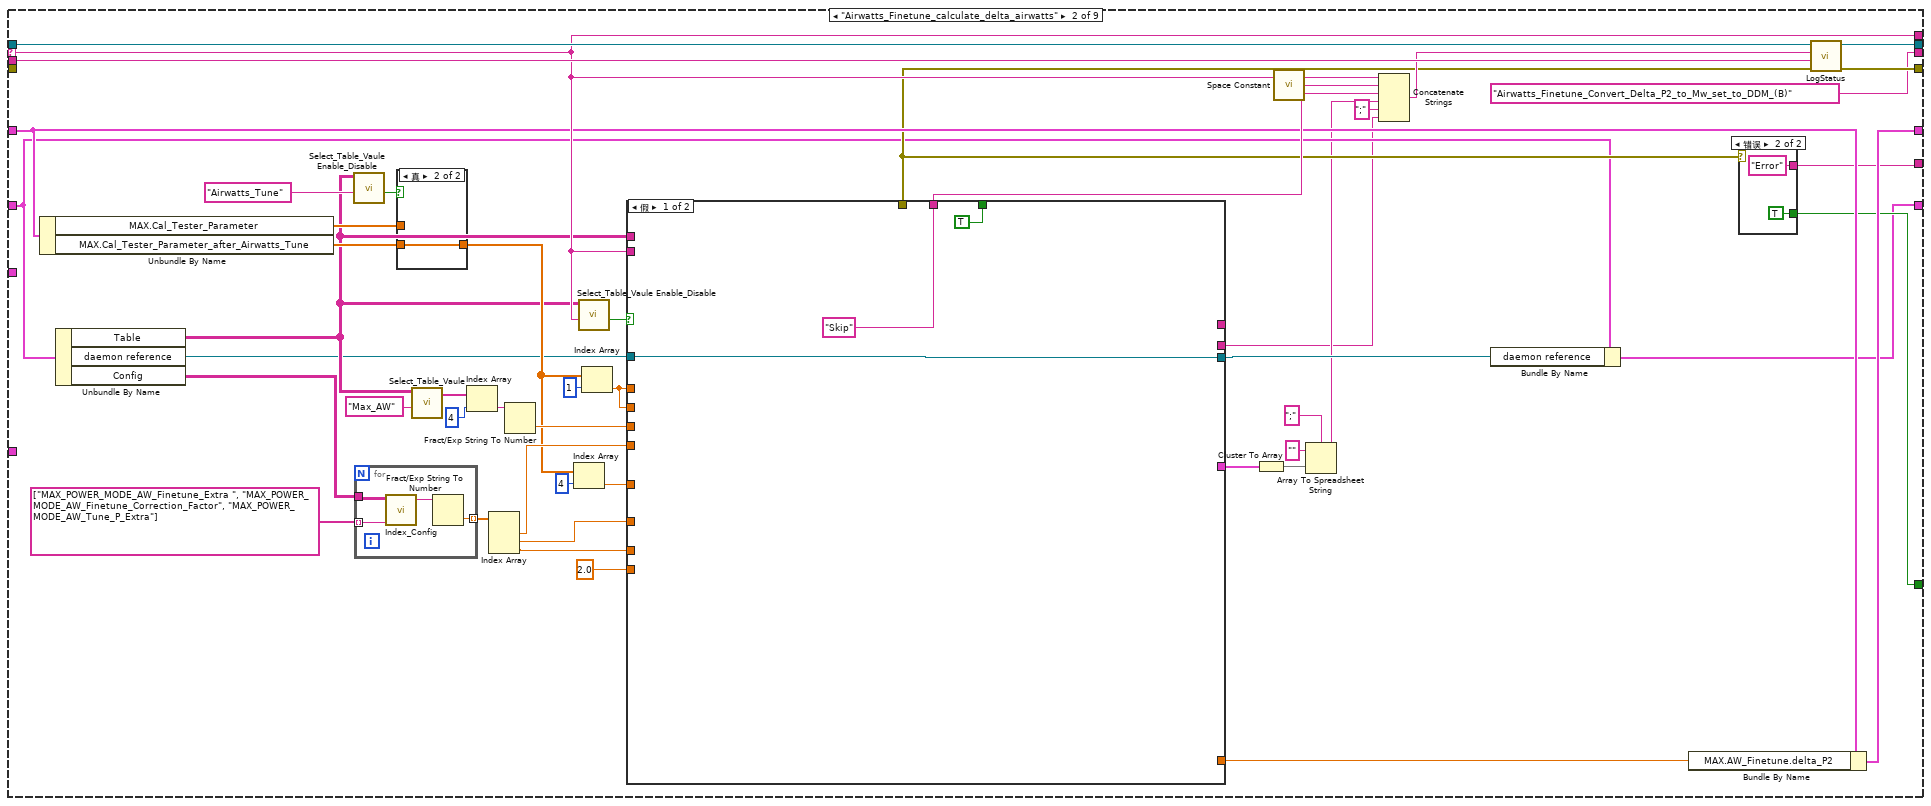
[diagram p3: hidden frame]
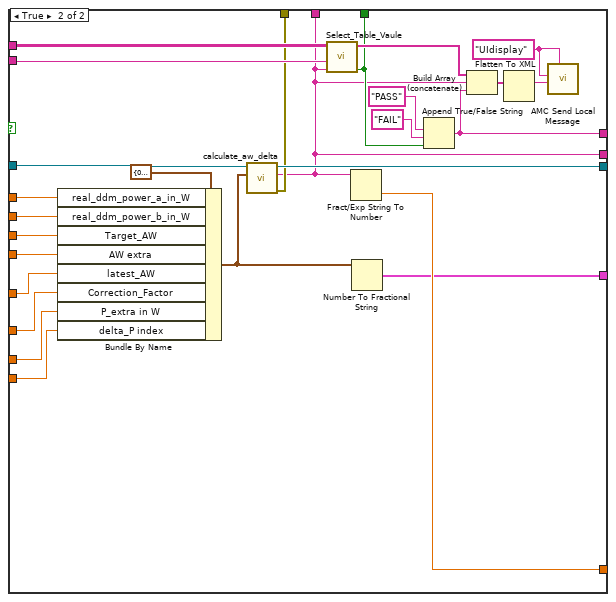
[diagram p6: hidden frame]
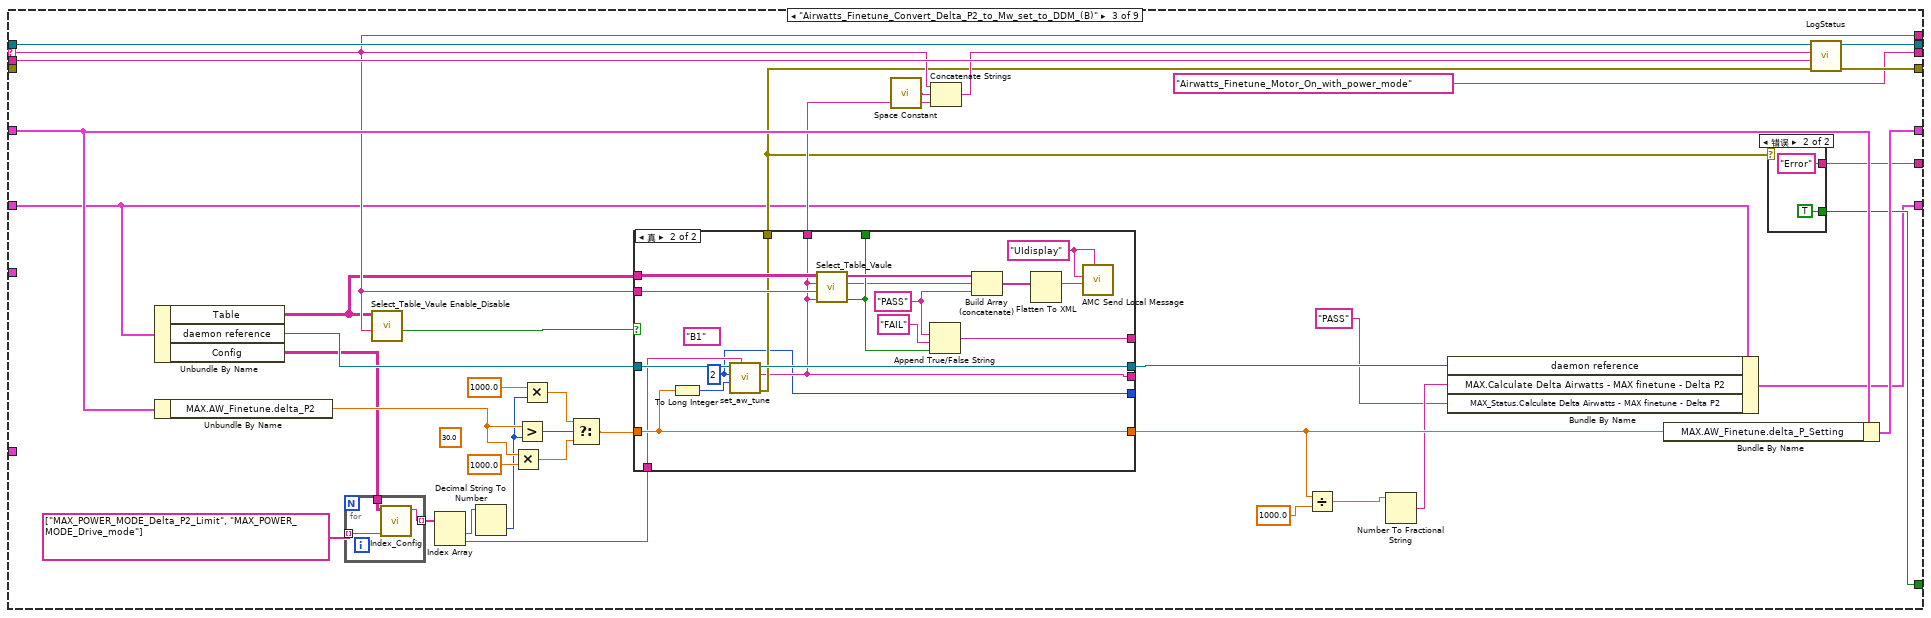
[diagram p7: hidden frame]
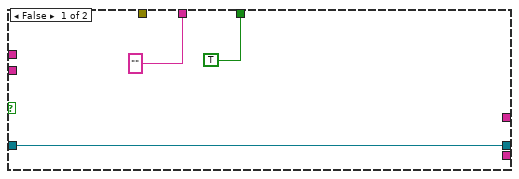
[diagram p9: hidden frame]
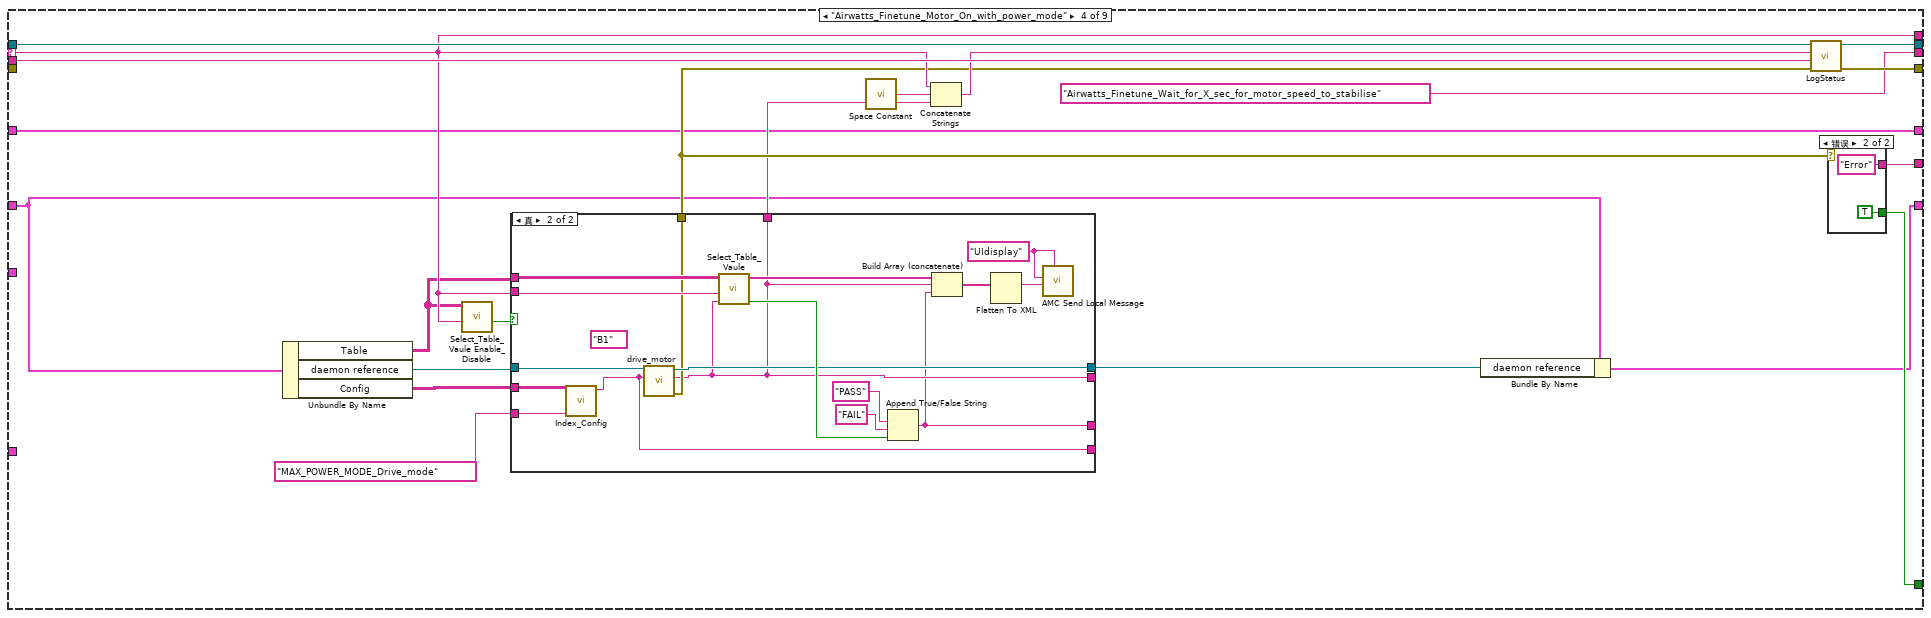
[diagram p10: hidden frame]
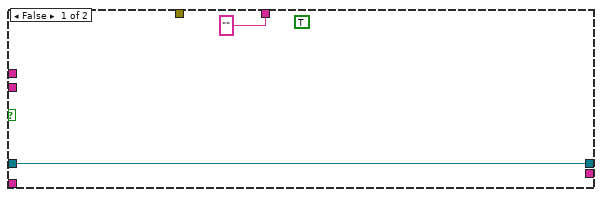
[diagram p12: hidden frame]
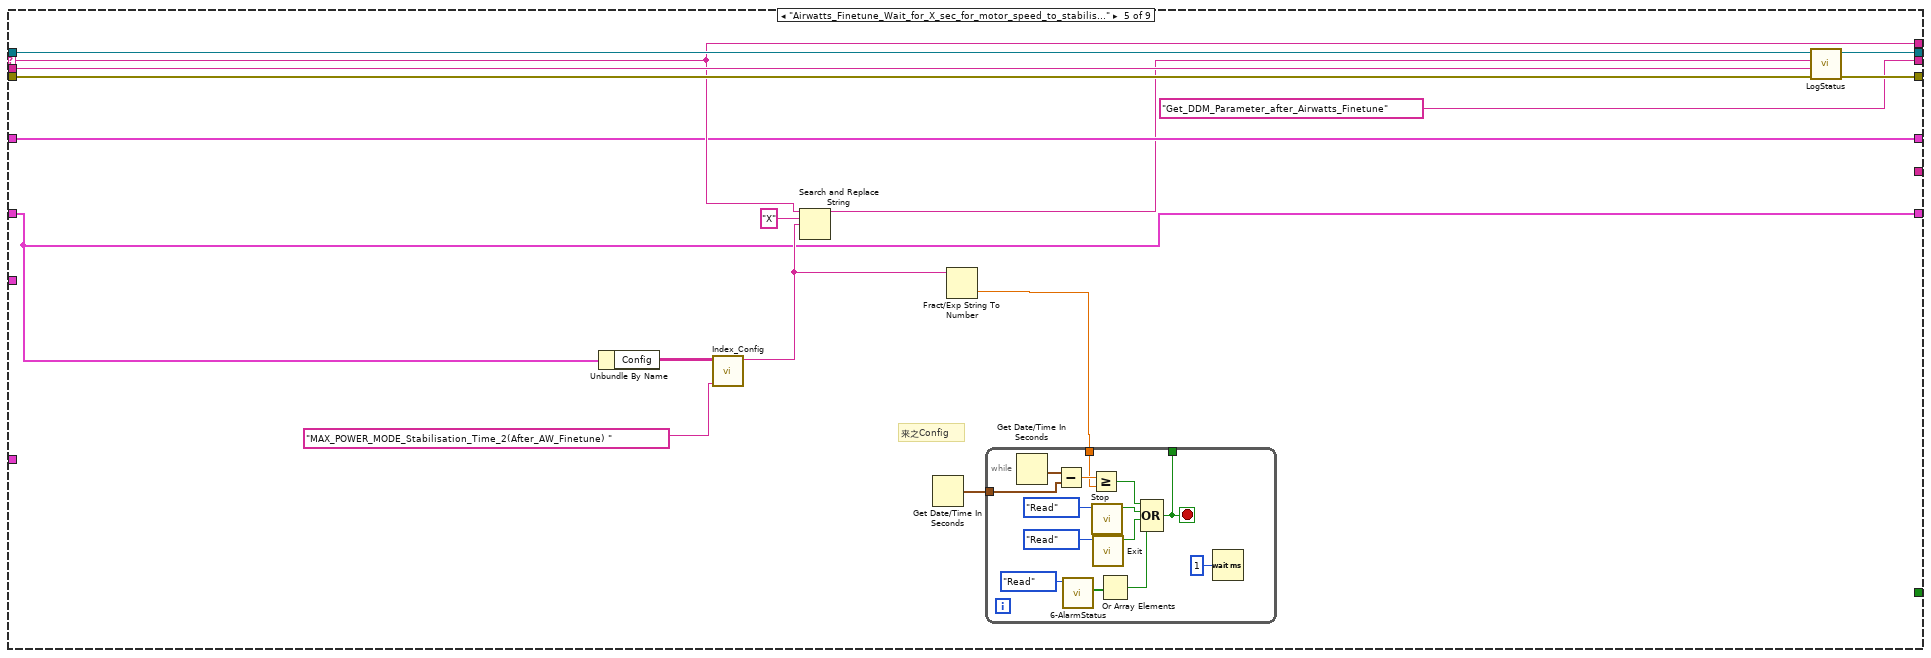
[diagram p13: hidden frame]
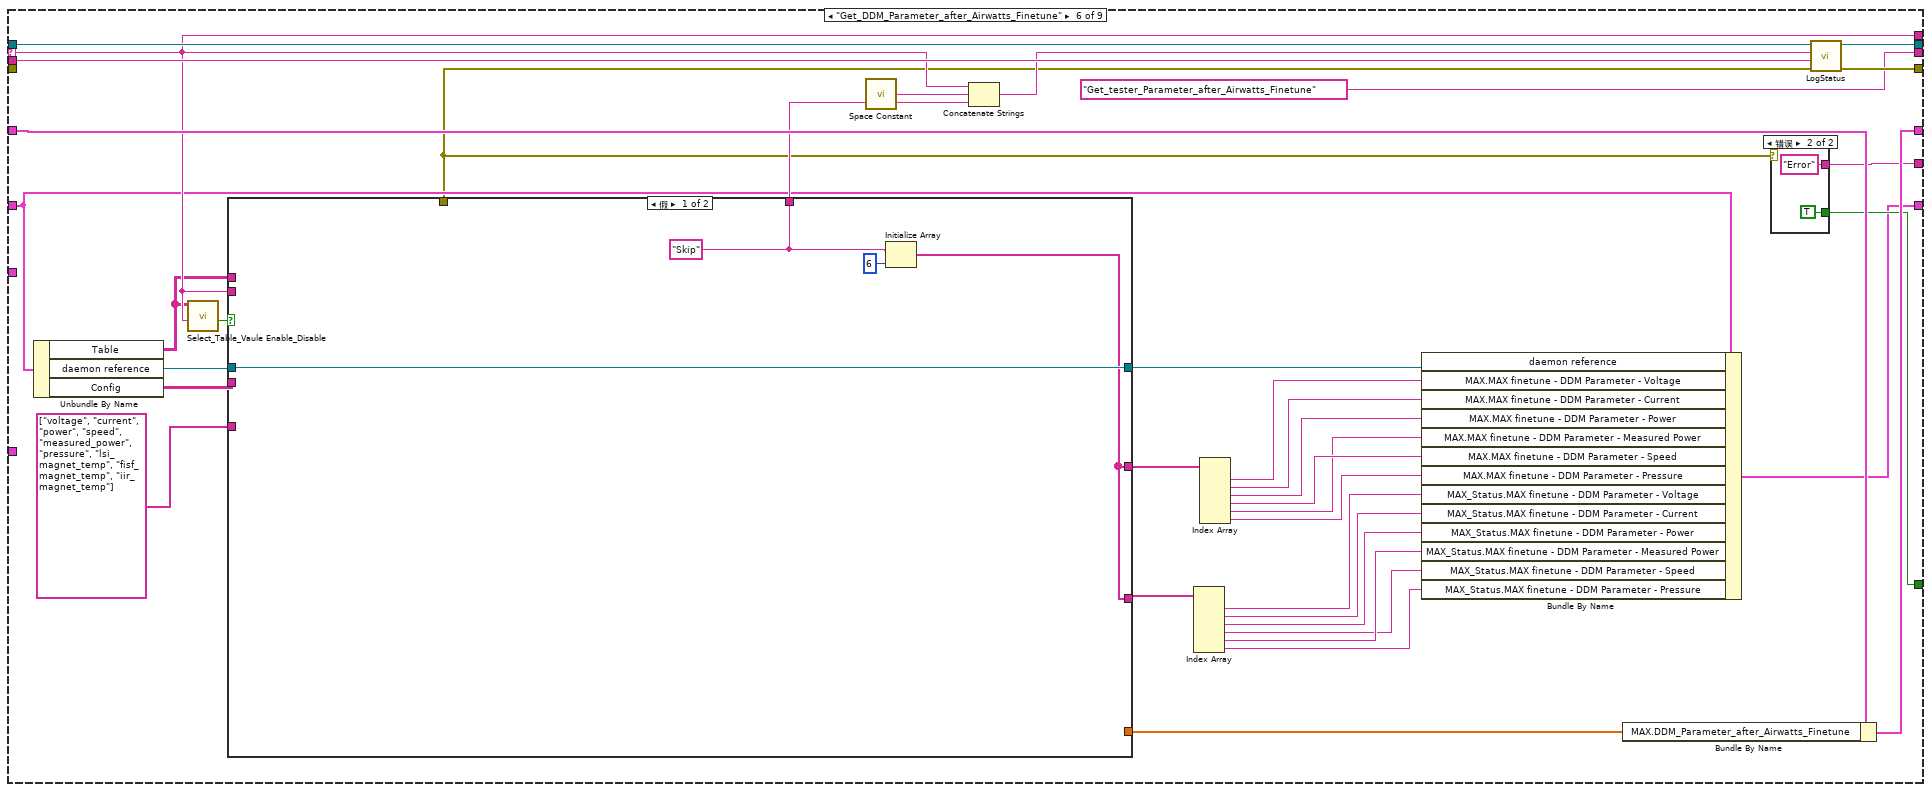
[diagram p14: hidden frame]
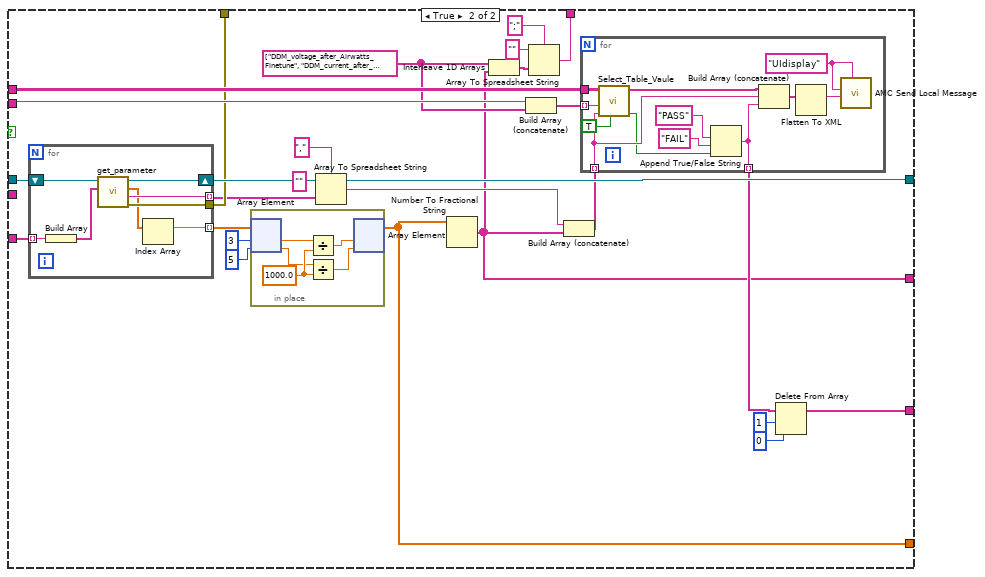
[diagram p16: hidden frame]
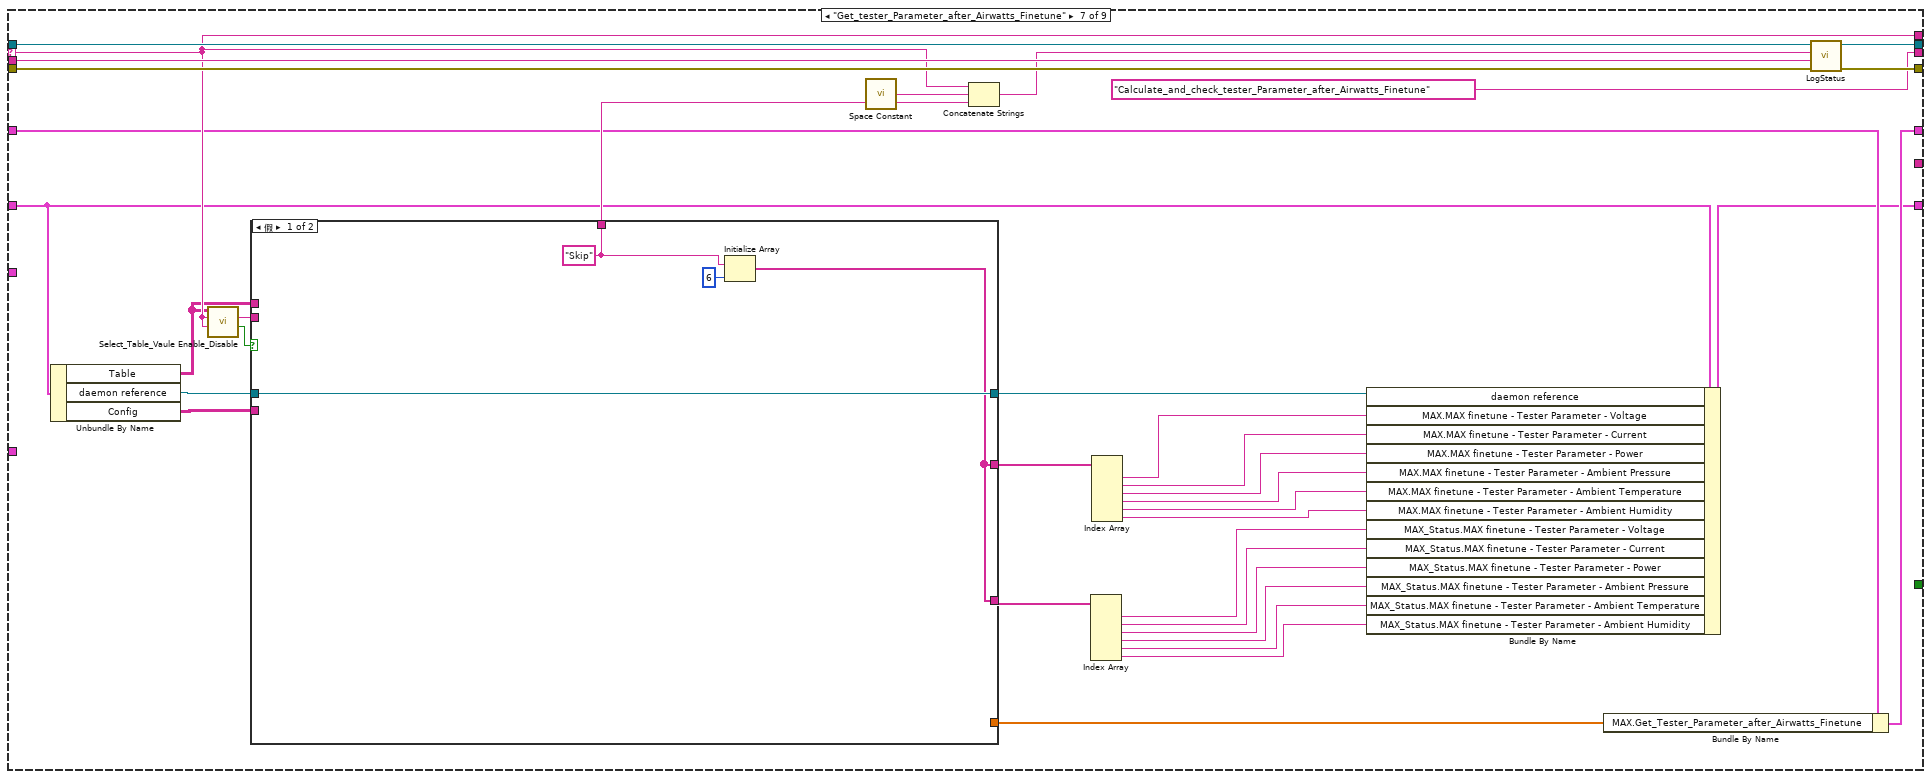
[diagram p17: hidden frame]
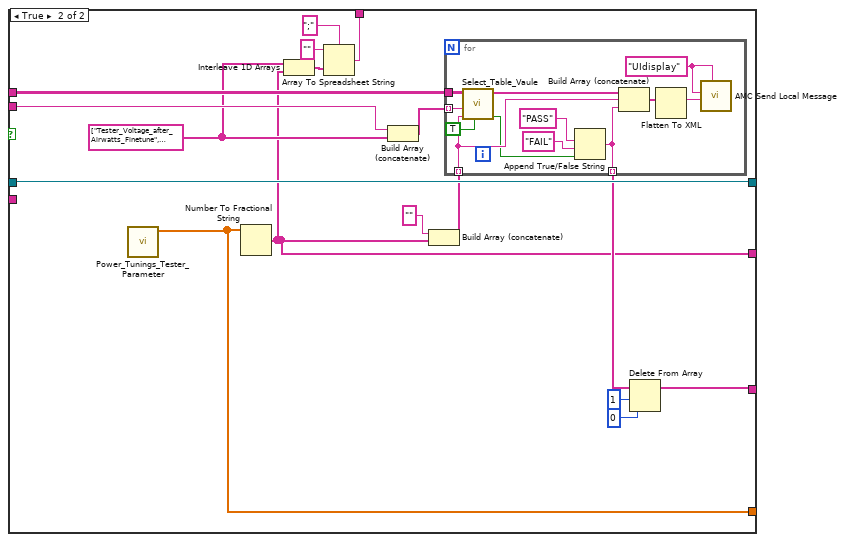
[diagram p18: hidden frame]
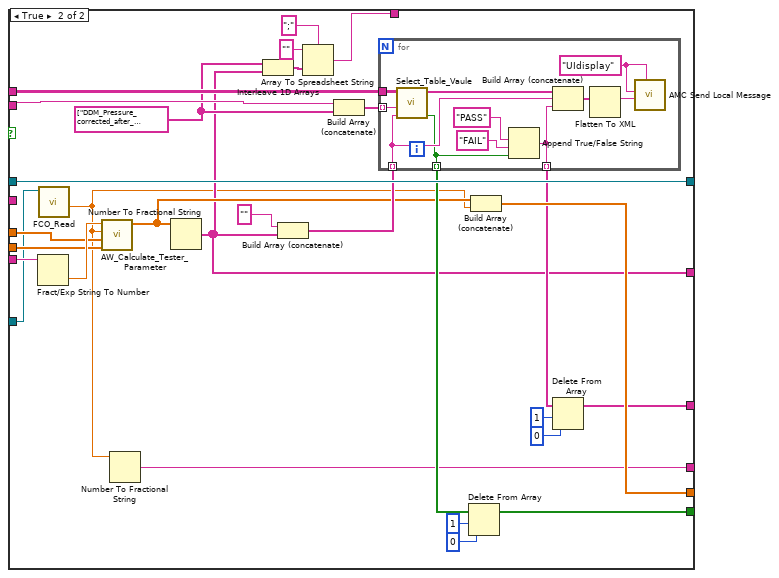
[diagram p19: hidden frame]
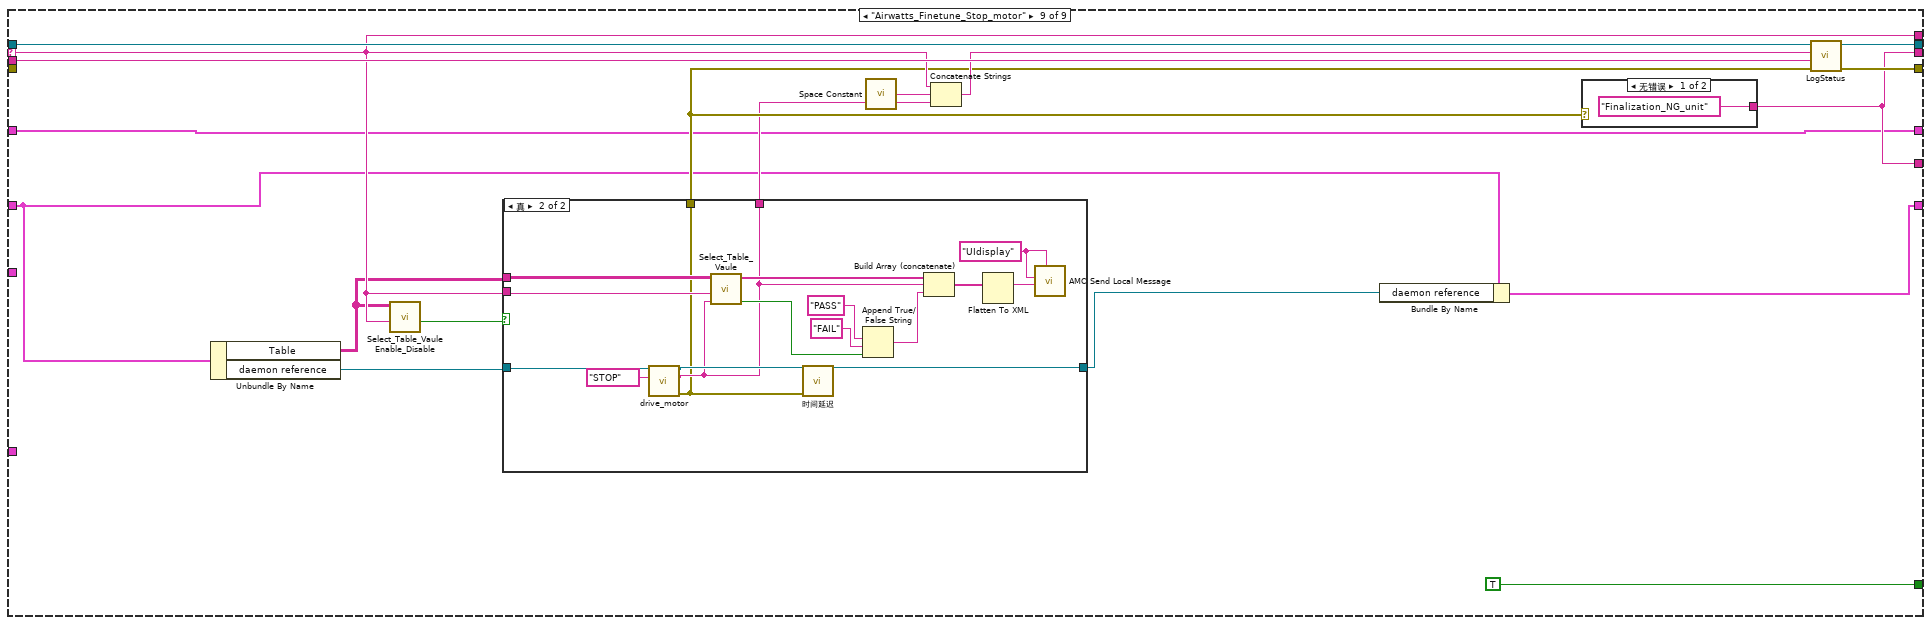
[diagram p20: hidden frame]
diagram:
  n1 = Flush Queue(queue="Message Queue out") -> (queue out=w4:T4)  [unwired: 1 in, 2 out]
  n2 = call "HD_Config.vi"("Step"=enum16{"Initial", "Write", "Read"}."Read") -> ("HD Config out"=w8:T5)  [unwired: 9 in, 1 out]
  n3 = call "AMC Send Local Message.vi"("error in (no error)"="error in (no error)", "Message Name"="Airwatts_Finetune_calculate_delta_airwatts", "Message Queue in"=w4) -> ("error out"=w13:errorcluster, "Message Queue out"=w14:T4)  [unwired: 7 in]
  n4 = while {
    tunnel: w14 -> [w47]
    tunnel: [w43] -> w6
    tunnel: w13 -> [w41]
    tunnel: [w38] -> w5
    shift-right: [w34] -> w10
    shift-left: "?" -> [w35]
    tunnel: w8 -> [w33]
    tunnel: [w29] -> w7
    shift-right: [w21] -> w1
    shift-left: "Data in" -> [w22]
    tunnel: "AllControls In" -> [w17]
    stop <- w23 stop-if-true
    n5 = Wait (ms)(milliseconds to wait=u32 1 ("等待时间（毫秒）")) -> ()  [unwired: 1 out]
    n6 = call "AMC Read Next Message.vi"("error in (no error)"=w41, "timeout (1ms)"=100, "Message Queue in"=w47) -> ("error out"=w40:errorcluster, "Message Value"=w31:string, "Message Name"=w45:string, "Message Queue out"=w46:T4)  [unwired: 1 in, 4 out]
    n7 = case shown="\"Calculate_and_check_tester_Parameter_after_Airwatts_Finetune\"" w45 {
      selector: w45 -> [_ w86 w164 w212 w250 w296 w386 w472 w535]
      tunnel: w46 -> [w51 w99 w173 w219 w255 w305 w395 w480 w541]
      tunnel: [w51 w99 w173 w219 w255 w305 w395 w480 w541] -> w44
      tunnel: w40 -> [w50 _ _ _ w254 _ w394 w479 _]
      tunnel: [w50 w98 w172 w218 w253 w304 w393 w478 w540] -> w39
      tunnel: [_ w71 w150 w206 _ w289 _ w429 TRUE ("Result")] -> w24
      tunnel: w35 -> [w49 w85 w170 w203 w249 w301 w381 w469 w526]
      tunnel: [w49 w88 w169 w203 w249 w300 w390 w476 w526] -> w34
      tunnel: w31 -> [_ w97 w171 w217 w252 w303 w392 w477 w539]
      tunnel: [_ w86 w164 w212 w250 w296 w386 w472 w535] -> w30
      tunnel: w33 -> [_ _ _ _ _ _ _ w460 _]
      tunnel: [_ "Airwatts_Finetune_Convert_Delta_P2_to_Mw_set_to_DDM_(B)" "Airwatts_Finetune_Motor_On_with_power_mode" "Airwatts_Finetune_Wait_for_X_sec_for_motor_speed_to_stabilise" "Get_DDM_Parameter_after_Airwatts_Finetune" ("t") "Get_tester_Parameter_after_Airwatts_Finetune" "Calculate_and_check_tester_Parameter_after_Airwatts_Finetune" w466 w532] -> w32
      tunnel: [_ w72 w151 w207 _ w290 _ w466 w532] -> w29
      tunnel: w22 -> [w48 w61 w145 w202 w241 w287 w379 w454 w528]
      tunnel: [w48 w60 w142 w200 w241 w286 w378 w453 w527] -> w21
      tunnel: w17 -> [_ _ _ _ _ _ _ w433 _]
      frame "假", Default {
      }
      frame "Airwatts_Finetune_calculate_delta_airwatts" {
        n8 = Unbundle By Name(w85) -> ("MAX.Cal_Tester_Parameter"=w67:dbl[], "MAX.Cal_Tester_Parameter_after_Airwatts_Tune"=w66:dbl[])
        n9 = Unbundle By Name(w61) -> ("Table"=w64:string[][], "daemon reference"=w63:refnum<k5>, "Config"=w62:string[][])
        n10 = call "Select_Table_Vaule Enable_Disable.vi"("Action"="Airwatts_Tune", "Table"=w64) -> ("Enable"=w68:bool)  [unwired: 8 in, 1 out]
        n11 = for {
          tunnel: w62 -> [w107]
          tunnel: string[] ["MAX_POWER_MODE_AW_Finetune_Extra ", "MAX_POWER_MODE_AW_Finetune_Correction_Factor", "MAX_POWER_MODE_AW_Tune_P_Extra"] -> [w106] mode=indexing
          tunnel: [w104] -> w77 mode=indexing
          n12 = call "Index_Config.vi"("Action"=w106, "config"=w107) -> ("data"=w105:string)  [unwired: 9 in]
          n13 = Fract/Exp String To Number(string=w105) -> (number=w104:dbl)  [unwired: 3 in, 1 out]
        }
        n14 = case shown="真" w68 {
          tunnel: w67 -> [w100 _]
          tunnel: w66 -> [_ w101]
          tunnel: [w100 w101] -> w65
          frame False {
          }
          frame True {
          }
        }
        n15 = call "Select_Table_Vaule.vi"("Action"="Max_AW", "Table"=w64) -> ("vaule"=w79:string[])  [unwired: 8 in, 1 out]
        n16 = Index Array(array=w79, index=4 ("索引")) -> (element=w81:string)
        n17 = Index Array(array=w77) -> (element #1=w75:dbl, element #2=w74:dbl, element #3=w73:dbl)  [unwired: 3 in]
        n18 = Fract/Exp String To Number(string=w81) -> (number=w78:dbl)  [unwired: 3 in, 1 out]
        n19 = Index Array(array=w65, index=4 ("索引")) -> (element=w91:dbl)
        n20 = call "Select_Table_Vaule Enable_Disable.vi"("Action"=w86, "Table"=w64) -> ("Enable"=w94:bool)  [unwired: 8 in, 1 out]
        n21 = Index Array(array=w65, index=1 ("索引")) -> (element=w84:dbl)
        n22 = case shown="假" w94 {
          tunnel: w63 -> [w109 w136]
          tunnel: [TRUE w126] -> _
          tunnel: [w109 w130] -> w59
          tunnel: ["Skip" ("response") w114] -> w87
          tunnel: w86 -> [_ w129]
          tunnel: w64 -> [_ w128]
          tunnel: w84 -> [_ w124]
          tunnel: w84 -> [_ w123]
          tunnel: w78 -> [_ w122]
          tunnel: w75 -> [_ w121]
          tunnel: w91 -> [_ w120]
          tunnel: w74 -> [_ w119]
          tunnel: w73 -> [_ w118]
          tunnel: 2.0 -> [_ w117]
          tunnel: [_ w116] -> w89
          tunnel: [_ w115] -> w70
          tunnel: [_ w114] -> w53
          tunnel: [_ w113] -> _
          tunnel: [_ w111] -> w58
          frame False {
          }
          frame True {
            w135 = "UIdisplay" ("Process (\"\" - local)")
            n23 = Bundle By Name(cluster=T6 {"real_ddm_power_a_in_W"=0.0, "real_ddm_power_b_in_W"=0.0, "Target_AW"=0.0, "AW extra"=0.0, "latest_AW"=0.0, "Correction_Factor"=0.0, "P_extra in W"=0.0, "delta_P index"=0.0} ("input"), "real_ddm_power_a_in_W"=w124, "real_ddm_power_b_in_W"=w123, "Target_AW"=w122, "AW extra"=w121, "latest_AW"=w120, "Correction_Factor"=w119, "P_extra in W"=w118, "delta_P index"=w117) -> (w112:T6)
            n24 = call "calculate_aw_delta.vi"("input"=w112, "daemon reference in"=w136) -> ("error out"=w115:errorcluster, "response"=w114:string, "daemon reference out"=w130:refnum<k5>)  [unwired: 6 in, 1 out]
            n25 = call "Select_Table_Vaule.vi"("Vaule"=w114, "Action"=w129, "Table"=w128) -> ("Result"=w126:bool, "vaule"=w127:string[])  [unwired: 7 in]
            n26 = Fract/Exp String To Number(string=w114) -> (number=w116:dbl)  [unwired: 3 in, 1 out]
            n27 = Number To Fractional String(number=w112) -> (F-format string=w111:T8)  [unwired: 3 in]
            n28 = Append True/False String(1:w126, 2:"FAIL" ("真字符串"), 3:"PASS" ("真字符串")) -> (0:w113:string)  [unwired: 1 in]
            n29 = Build Array (concatenate)(w127, w114, w113) -> (w134:string[])
            n30 = Flatten To XML(anything=w134) -> (xml string=w133:string)
            n31 = call "AMC Send Local Message.vi"("Process (\"\" - local)"=w135, "Message Value"=w133, "Message Name"=w135) -> ()  [unwired: 7 in, 2 out]
          }
        }
        n32 = Cluster To Array(cluster=w58) -> (array=w57:string[])
        n33 = call <vilib>:"Space Constant.vi"() -> ("String"=w96:string)
        n34 = Array To Spreadsheet String(delimiter (Tab)=";" ("分隔符(Tab)"), array=w57, 3:"" ("格式字符串")) -> (spreadsheet string=w54:string)
        n35 = Concatenate Strings(w86, w96, w87, w54, ";" ("字符串"), w53) -> (w95:string)
        n36 = Bundle By Name(cluster=w61, "daemon reference"=w59) -> (w60:T1)
        n37 = Bundle By Name(cluster=w85, "MAX.AW_Finetune.delta_P2"=w89) -> (w88:T3)
        n38 = case shown="错误" w70 {
          tunnel: [_ TRUE] -> w71
          tunnel: [_ "Error"] -> w72
          frame No Error {
          }
          frame Error {
          }
        }
        n39 = call "LogStatus.vi"("error in (no error)"=w70, "last message"=w97, "message"=w95) -> ("error  out"=w98:errorcluster)  [unwired: 8 in]
      }
      frame "Airwatts_Finetune_Convert_Delta_P2_to_Mw_set_to_DDM_(B)" {
        (unwired) 30.0 ("y")
        n40 = Unbundle By Name(w145) -> ("Table"=w148:string[][], "daemon reference"=w147:refnum<k5>, "Config"=w146:string[][])
        n41 = Unbundle By Name(w170) -> ("MAX.AW_Finetune.delta_P2"=w158:dbl)
        n42 = for {
          tunnel: w146 -> [w178]
          tunnel: string[] ["MAX_POWER_MODE_Delta_P2_Limit", "MAX_POWER_MODE_Drive_mode"] -> [w177] mode=indexing
          tunnel: [w176] -> w155 mode=indexing
          n43 = call "Index_Config.vi"("Action"=w177, "config"=w178) -> ("data"=w176:string)  [unwired: 9 in]
        }
        n44 = call "Select_Table_Vaule Enable_Disable.vi"("Action"=w164, "Table"=w148) -> ("Enable"=w165:bool)  [unwired: 8 in, 1 out]
        n45 = Index Array(array=w155) -> (element #1=w154:string, element #2=w144:string)  [unwired: 2 in]
        n46 = Decimal String To Number(string=w154) -> (number=w153:i32)  [unwired: 2 in, 1 out]
        n47 = Multiply(x=w158, y=1000.0) -> (x*y=w162:dbl)
        n48 = Greater?(x=w158, y=w153) -> (0:w161:bool)
        n49 = Multiply(x=1000.0 ("y"), y=w153) -> (x*y=w163:dbl)
        n50 = Select(t=w163, s=w161, f=w162) -> (s? t:f=w157:dbl)
        n51 = case shown="真" w165 {
          tunnel: w147 -> [w180 w190]
          tunnel: [TRUE w192] -> _
          tunnel: [w180 w189] -> w143
          tunnel: ["" ("software string") w185] -> w166
          tunnel: w164 -> [_ w195]
          tunnel: w148 -> [_ w194]
          tunnel: w157 -> [_ w188]
          tunnel: [_ w188] -> w139
          tunnel: w144 -> [_ w187]
          tunnel: [_ w186] -> w149
          tunnel: [_ w185] -> _
          tunnel: [_ w184] -> _
          tunnel: [_ w183] -> _
          frame False {
          }
          frame True {
            (unwired) "B1" ("Power Mode or Target Power in W")
            w183 = 2 ("Index")
            w182 = "PASS" ("真字符串")
            w199 = "UIdisplay" ("Process (\"\" - local)")
            n52 = To Long Integer(number=w188) -> (32bit integer=w191:i32)
            n53 = call "set_aw_tune.vi"("Power Mode or Target Power in W"=w187, "Offset Power mW"=w191, "Index"=w183, "daemon reference in"=w190) -> ("error out"=w186:errorcluster, "response"=w185:string, "daemon reference out"=w189:refnum<k5>)  [unwired: 4 in, 1 out]
            n54 = call "Select_Table_Vaule.vi"("Vaule"=w185, "Action"=w195, "Table"=w194) -> ("Result"=w192:bool, "vaule"=w193:string[])  [unwired: 7 in]
            n55 = Append True/False String(1:w192, 2:"FAIL" ("真字符串"), 3:w182) -> (0:w184:string)  [unwired: 1 in]
            n56 = Build Array (concatenate)(w193, w185, w182) -> (w198:string[])
            n57 = Flatten To XML(anything=w198) -> (xml string=w197:string)
            n58 = call "AMC Send Local Message.vi"("Process (\"\" - local)"=w199, "Message Value"=w197, "Message Name"=w199) -> ()  [unwired: 7 in, 2 out]
          }
        }
        n59 = call <vilib>:"Space Constant.vi"() -> ("String"=w168:string)
        n60 = Concatenate Strings(w164, w168, w166) -> (w167:string)
        n61 = Divide(x=w139, y=1000.0) -> (x/y=w140:dbl)
        n62 = Number To Fractional String ("数值至小数字符串转换")(number=w140) -> (F-format string=w138:string)  [unwired: 3 in]
        n63 = Bundle By Name(cluster=w145, "daemon reference"=w143, "MAX.Calculate Delta Airwatts - MAX finetune - Delta P2"=w138, "MAX_Status.Calculate Delta Airwatts - MAX finetune - Delta P2"="PASS" ("真字符串")) -> (w142:T1)
        n64 = Bundle By Name(cluster=w170, "MAX.AW_Finetune.delta_P_Setting"=w139) -> (w169:T3)
        n65 = case shown="错误" w149 {
          tunnel: [_ TRUE] -> w150
          tunnel: [_ "Error"] -> w151
          frame No Error {
          }
          frame Error {
          }
        }
        n66 = call "LogStatus.vi"("error in (no error)"=w149, "last message"=w171, "message"=w167) -> ("error  out"=w172:errorcluster)  [unwired: 8 in]
      }
      frame "Airwatts_Finetune_Motor_On_with_power_mode" {
        n67 = Unbundle By Name(w202) -> ("Table"=w211:string[][], "daemon reference"=w216:refnum<k5>, "Config"=w209:string[][])
        n68 = call "Select_Table_Vaule Enable_Disable.vi"("Action"=w212, "Table"=w211) -> ("Enable"=w210:bool)  [unwired: 8 in, 1 out]
        n69 = case shown="真" w210 {
          tunnel: w216 -> [w223 w231]
          tunnel: [w223 w230] -> w201
          tunnel: ["" ("software string") w226] -> w204
          tunnel: w212 -> [_ w235]
          tunnel: w211 -> [_ w234]
          tunnel: w209 -> [_ w229]
          tunnel: "MAX_POWER_MODE_Drive_mode" -> [_ w228]
          tunnel: [_ w227] -> w205
          tunnel: [_ w226] -> _
          tunnel: [_ w225] -> _
          tunnel: [_ w224] -> _
          frame False {
            (unwired) TRUE
          }
          frame True {
            (unwired) "B1" ("Power Mode")
            w240 = "UIdisplay" ("Process (\"\" - local)")
            n70 = call "Index_Config.vi"("Action"=w228, "config"=w229) -> ("data"=w224:string)  [unwired: 9 in]
            n71 = call "drive_motor.vi"("Power Mode"=w224, "daemon reference in"=w231) -> ("error out"=w227:errorcluster, "response"=w226:string, "daemon reference out"=w230:refnum<k5>)  [unwired: 6 in, 1 out]
            n72 = call "Select_Table_Vaule.vi"("Vaule"=w226, "Action"=w235, "Table"=w234) -> ("Result"=w232:bool, "vaule"=w233:string[])  [unwired: 7 in]
            n73 = Append True/False String(1:w232, 2:"FAIL" ("真字符串"), 3:"PASS" ("真字符串")) -> (0:w225:string)  [unwired: 1 in]
            n74 = Build Array (concatenate)(w233, w226, w225) -> (w239:string[])
            n75 = Flatten To XML(anything=w239) -> (xml string=w238:string)
            n76 = call "AMC Send Local Message.vi"("Process (\"\" - local)"=w240, "Message Value"=w238, "Message Name"=w240) -> ()  [unwired: 7 in, 2 out]
          }
        }
        n77 = call <vilib>:"Space Constant.vi"() -> ("String"=w215:string)
        n78 = Concatenate Strings(w212, w215, w204) -> (w214:string)
        n79 = Bundle By Name(cluster=w202, "daemon reference"=w201) -> (w200:T1)
        n80 = call "LogStatus.vi"("error in (no error)"=w205, "last message"=w217, "message"=w214) -> ("error  out"=w218:errorcluster)  [unwired: 8 in]
        n81 = case shown="错误" w205 {
          tunnel: [_ TRUE] -> w206
          tunnel: [_ "Error"] -> w207
          frame No Error {
          }
          frame Error {
          }
        }
      }
      frame "Airwatts_Finetune_Wait_for_X_sec_for_motor_speed_to_stabilise" {
        # "来之Config"
        n82 = Unbundle By Name(w241) -> ("Config"=w246:string[][])
        n83 = call "Index_Config.vi"("Action"="MAX_POWER_MODE_Stabilisation_Time_2(After_AW_Finetune) ", "config"=w246) -> ("data"=w244:string)  [unwired: 9 in]
        n84 = Search and Replace String(input string=w250, search string="X" ("搜索字符串"), replace string=w244) -> (result string=w248:string)  [unwired: 5 in, 3 out]
        n85 = Get Date/Time In Seconds() -> (seconds since 1Jan1904=w243:timestamp)
        n86 = Fract/Exp String To Number(string=w244) -> (number=w242:dbl)  [unwired: 3 in, 1 out]
        n87 = while {
          tunnel: w243 -> [w262]
          tunnel: w242 -> [w259]
          tunnel: [w258] -> _
          stop <- w258 stop-if-true
          n88 = Get Date/Time In Seconds() -> (seconds since 1Jan1904=w263:timestamp)
          n89 = Subtract(x=w263, y=w262) -> (x-y=w261:dbl)
          n90 = call "6-AlarmStatus.vi"("Step"=enum16{"Initial", "Write", "Read"}."Read") -> ("AlarmValue Out"=w266:bool[])  [unwired: 9 in, 1 out]
          n91 = Greater Or Equal?(x=w261, y=w259) -> (x >= y?=w260:bool)
          n92 = call "Stop.vi"("Step"=enum16{"Initial", "Write", "Read"}."Read") -> ("Stop Out"=w264:bool)  [unwired: 9 in, 1 out]
          n93 = call "Exit.vi"("Step"=enum16{"Initial", "Write", "Read"}."Read" ("step")) -> ("Exit Out"=w268:bool)  [unwired: 9 in, 1 out]
          n94 = Or Array Elements(Boolean array=w266) -> (logical OR=w265:bool)
          n95 = Compound Arithmetic op=OR(w260, w264, w268, w265) -> (w258:bool)
          n96 = Wait (ms)(milliseconds to wait=u32 1 ("等待时间（毫秒）")) -> ()  [unwired: 1 out]
        }
        n97 = call "LogStatus.vi"("error in (no error)"=w254, "last message"=w252, "message"=w248) -> ("error  out"=w253:errorcluster)  [unwired: 8 in]
      }
      frame "Get_DDM_Parameter_after_Airwatts_Finetune" {
        n98 = Unbundle By Name(w287) -> ("Table"=w295:string[][], "daemon reference"=w302:refnum<k5>, "Config"=w293:string[][])
        n99 = call "Select_Table_Vaule Enable_Disable.vi"("Action"=w296, "Table"=w295) -> ("Enable"=w294:bool)  [unwired: 8 in, 1 out]
        n100 = case shown="假" w294 {
          tunnel: w302 -> [w311 w336]
          tunnel: [w311 w335] -> w283
          tunnel: [w310 w328] -> w297
          tunnel: w296 -> [_ w334]
          tunnel: w295 -> [_ w337]
          tunnel: w293 -> [_ _]
          tunnel: [_ w322] -> w291
          tunnel: [_ w326] -> w284
          tunnel: T7[] ["voltage", "current", "power", "speed", "measured_power", "pressure", "lsi_magnet_temp", "fisf_magnet_temp", "iir_magnet_temp"] ("Parameter") -> [_ w321]
          tunnel: [w309 w313] -> w276
          tunnel: [w309 w312] -> w285
          frame False {
            w310 = "Skip" ("software string")
            n101 = Initialize Array(w310, 6 ("维数大小")) -> (w309:string[])
          }
          frame True {
            w327 = string[] ["DDM_voltage_after_Airwatts_Finetune", "DDM_current_after_Airwatts_Finetune", "DDM_power_after_Airwatts_Finetune", "DDM_speed_after_Airwatts_Finetune", "DDM_measured_power_after_Airwatts_Finetune", "DDM_pressure_after_Airwatts_Finetune", "DDM_lsi_magnet_temp_after_Airwatts_Finetune", "DDM_fisf_magnet_temp_after_Airwatts_Finetune", "DDM_iir_magnet_temp_after_Airwatts_Finetune"]
            n102 = for {
              tunnel: [w343] -> w320 mode=indexing
              tunnel: [w342] -> w326
              tunnel: [w338] -> w323 mode=indexing
              tunnel: w321 -> [w340] mode=indexing
              shift-right: [w344] -> w335
              shift-left: w336 -> [w345]
              n103 = Build Array(w340) -> (w339:T7[])
              n104 = call "get_parameter.vi"("Parameter"=w339, "daemon reference in"=w345) -> ("error out"=w342:errorcluster, "response"=w343:string, "values"=w341:dbl[], "daemon reference out"=w344:refnum<k5>)  [unwired: 5 in, 1 out]
              n105 = Index Array(array=w341) -> (element=w338:dbl)  [unwired: 1 in]
            }
            n106 = in-place {
              w350 = 1000.0
              n107 = in-place-array #1(w323, 3, 5) -> (w349:dbl, w346:dbl)
              n108 = Divide(x=w349, y=w350) -> (x/y=w348:dbl)
              n109 = Divide(x=w346, y=w350) -> (x/y=w347:dbl)
              n110 = in-place-array #1(w348, w347) -> (w322:dbl[])  [unwired: 2 out]
            }
            n111 = Array To Spreadsheet String(delimiter (Tab)=",", array=w320, 3:"" ("format string")) -> (spreadsheet string=w319:string)
            n112 = Number To Fractional String(number=w322) -> (F-format string=w312:string[])  [unwired: 3 in]
            n113 = Interleave 1D Arrays(w327, w312) -> (w329:string[])
            n114 = Build Array (concatenate)(w334, w327) -> (w333:string[])
            n115 = Array To Spreadsheet String(delimiter (Tab)=";" ("分隔符(Tab)"), array=w329, 3:"" ("格式字符串")) -> (spreadsheet string=w328:string)
            n116 = Build Array (concatenate)(w319, w312) -> (w332:string[])
            n117 = for {
              tunnel: w337 -> [w357]
              tunnel: w332 -> [w355] mode=indexing
              tunnel: w333 -> [w354] mode=indexing
              tunnel: [w351] -> w314 mode=indexing
              w362 = "UIdisplay" ("Process (\"\" - local)")
              n118 = call "Select_Table_Vaule.vi"("Boolean"=TRUE, "Vaule"=w355, "Action"=w354, "Table"=w357) -> ("Result"=w353:bool, "vaule"=w356:string[])  [unwired: 6 in]
              n119 = Append True/False String(1:w353, 2:"FAIL" ("真字符串"), 3:"PASS" ("真字符串")) -> (0:w351:string)  [unwired: 1 in]
              n120 = Build Array (concatenate)(w356, w355, w351) -> (w361:string[])
              n121 = Flatten To XML(anything=w361) -> (xml string=w360:string)
              n122 = call "AMC Send Local Message.vi"("Process (\"\" - local)"=w362, "Message Value"=w360, "Message Name"=w362) -> ()  [unwired: 7 in, 2 out]
            }
            n123 = Delete From Array(array=w314, length=1, index=0) -> (array with subset deleted=w313:string[])  [unwired: 1 out]
          }
        }
        n124 = call <vilib>:"Space Constant.vi"() -> ("String"=w299:string)
        n125 = Concatenate Strings(w296, w299, w297) -> (w298:string)
        n126 = Index Array(array=w276) -> (element #1=w275:string, element #2=w274:string, element #3=w273:string, element #4=w271:string, element #5=w272:string, element #6=w270:string)  [unwired: 6 in]
        n127 = Index Array(array=w285) -> (element #1=w282:string, element #2=w281:string, element #3=w280:string, element #4=w279:string, element #5=w278:string, element #6=w277:string)  [unwired: 6 in]
        n128 = Bundle By Name(cluster=w287, "daemon reference"=w283, "MAX.MAX finetune - DDM Parameter - Voltage"=w282, "MAX.MAX finetune - DDM Parameter - Current"=w281, "MAX.MAX finetune - DDM Parameter - Power"=w280, "MAX.MAX finetune - DDM Parameter - Measured Power"=w278, "MAX.MAX finetune - DDM Parameter - Speed"=w279, "MAX.MAX finetune - DDM Parameter - Pressure"=w277, "MAX_Status.MAX finetune - DDM Parameter - Voltage"=w275, "MAX_Status.MAX finetune - DDM Parameter - Current"=w274, "MAX_Status.MAX finetune - DDM Parameter - Power"=w273, "MAX_Status.MAX finetune - DDM Parameter - Measured Power"=w272, "MAX_Status.MAX finetune - DDM Parameter - Speed"=w271, "MAX_Status.MAX finetune - DDM Parameter - Pressure"=w270) -> (w286:T1)
        n129 = Bundle By Name(cluster=w301, "MAX.DDM_Parameter_after_Airwatts_Finetune"=w291) -> (w300:T3)
        n130 = case shown="错误" w284 {
          tunnel: [_ TRUE] -> w289
          tunnel: [_ "Error"] -> w290
          frame No Error {
          }
          frame Error {
          }
        }
        n131 = call "LogStatus.vi"("error in (no error)"=w284, "last message"=w303, "message"=w298) -> ("error  out"=w304:errorcluster)  [unwired: 8 in]
      }
      frame "Get_tester_Parameter_after_Airwatts_Finetune" {
        n132 = Unbundle By Name(w379) -> ("Table"=w385:string[][], "daemon reference"=w391:refnum<k5>, "Config"=w383:string[][])
        n133 = call "Select_Table_Vaule Enable_Disable.vi"("Action"=w386, "Table"=w385) -> ("Enable"=w384:bool)  [unwired: 8 in, 1 out]
        n134 = case shown="假" w384 {
          tunnel: w391 -> [w399 w415]
          tunnel: [w399 w415] -> w376
          tunnel: [w398 w407] -> w387
          tunnel: w386 -> [_ w413]
          tunnel: w385 -> [_ w416]
          tunnel: w383 -> [_ _]
          tunnel: [_ w405] -> w382
          tunnel: [w397 w401] -> w377
          tunnel: [w397 w400] -> w369
          frame False {
            w398 = "Skip" ("software string")
            n135 = Initialize Array(w398, 6 ("维数大小")) -> (w397:string[])
          }
          frame True {
            w406 = string[] ["Tester_Voltage_after_Airwatts_Finetune", "Tester_Current_after_Airwatts_Finetune", "Tester_Power_after_Airwatts_Finetune", "Tester_Ambient_Pressure_after_Airwatts_Finetune", "Tester_Ambient_Temperature_after_Airwatts_Finetune", "Tester_Ambient_humidity_after_Airwatts_Finetune", "Tester_Reference_Ambient_Pressure_after_Airwatts_Finetune"]
            n136 = call "Power_Tunings_Tester_Parameter.vi"() -> ("Power_Tuning_Tester_Parameter"=w405:dbl[])  [unwired: 11 in]
            n137 = Number To Fractional String(number=w405) -> (F-format string=w401:string[])  [unwired: 3 in]
            n138 = Interleave 1D Arrays(w406, w401) -> (w408:string[])
            n139 = Array To Spreadsheet String(delimiter (Tab)=";" ("分隔符(Tab)"), array=w408, 3:"" ("格式字符串")) -> (spreadsheet string=w407:string)
            n140 = Build Array (concatenate)(w413, w406) -> (w414:string[])
            n141 = Build Array (concatenate)("", w401) -> (w412:string[])
            n142 = for {
              tunnel: w416 -> [w423]
              tunnel: w412 -> [w421] mode=indexing
              tunnel: w414 -> [w420] mode=indexing
              tunnel: [w417] -> w402 mode=indexing
              w428 = "UIdisplay" ("Process (\"\" - local)")
              n143 = call "Select_Table_Vaule.vi"("Boolean"=TRUE, "Vaule"=w421, "Action"=w420, "Table"=w423) -> ("Result"=w419:bool, "vaule"=w422:string[])  [unwired: 6 in]
              n144 = Append True/False String(1:w419, 2:"FAIL" ("真字符串"), 3:"PASS" ("真字符串")) -> (0:w417:string)  [unwired: 1 in]
              n145 = Build Array (concatenate)(w422, w421, w417) -> (w427:string[])
              n146 = Flatten To XML(anything=w427) -> (xml string=w426:string)
              n147 = call "AMC Send Local Message.vi"("Process (\"\" - local)"=w428, "Message Value"=w426, "Message Name"=w428) -> ()  [unwired: 7 in, 2 out]
            }
            n148 = Delete From Array(array=w402, length=1, index=0) -> (array with subset deleted=w400:string[])  [unwired: 1 out]
          }
        }
        n149 = call <vilib>:"Space Constant.vi"() -> ("String"=w389:string)
        n150 = Concatenate Strings(w386, w389, w387) -> (w388:string)
        n151 = Index Array(array=w369) -> (element #1=w368:string, element #2=w367:string, element #3=w366:string, element #4=w365:string, element #5=w364:string, element #6=w363:string)  [unwired: 6 in]
        n152 = Index Array(array=w377) -> (element #1=w375:string, element #2=w374:string, element #3=w373:string, element #4=w372:string, element #5=w371:string, element #6=w370:string)  [unwired: 6 in]
        n153 = Bundle By Name(cluster=w379, "daemon reference"=w376, "MAX.MAX finetune - Tester Parameter - Voltage"=w375, "MAX.MAX finetune - Tester Parameter - Current"=w374, "MAX.MAX finetune - Tester Parameter - Power"=w373, "MAX.MAX finetune - Tester Parameter - Ambient Pressure"=w372, "MAX.MAX finetune - Tester Parameter - Ambient Temperature"=w371, "MAX.MAX finetune - Tester Parameter - Ambient Humidity"=w370, "MAX_Status.MAX finetune - Tester Parameter - Voltage"=w368, "MAX_Status.MAX finetune - Tester Parameter - Current"=w367, "MAX_Status.MAX finetune - Tester Parameter - Power"=w366, "MAX_Status.MAX finetune - Tester Parameter - Ambient Pressure"=w365, "MAX_Status.MAX finetune - Tester Parameter - Ambient Temperature"=w364, "MAX_Status.MAX finetune - Tester Parameter - Ambient Humidity"=w363) -> (w378:T1)
        n154 = Bundle By Name(cluster=w381, "MAX.Get_Tester_Parameter_after_Airwatts_Finetune"=w382) -> (w390:T3)
        n155 = call "LogStatus.vi"("error in (no error)"=w394, "last message"=w392, "message"=w388) -> ("error  out"=w393:errorcluster)  [unwired: 8 in]
      }
      frame "Calculate_and_check_tester_Parameter_after_Airwatts_Finetune" {
        n156 = Unbundle By Name(w469) -> ("MAX.DDM_Parameter_after_Airwatts_Finetune"=w464:dbl[], "MAX.Get_Tester_Parameter_after_Airwatts_Finetune"=w463:dbl[])
        n157 = Unbundle By Name(w454) -> ("Table"=w457:string[][], "daemon reference"=w456:refnum<k5>, "Config"=w455:string[][])
        n158 = Unbundle By Name(w460) -> ("FCO.COM"=w461:refnum<visa-resource-name>)
        n159 = call "Index_Config.vi"("Action"="MAX_POWER_MODE_Orifice_size", "config"=w455) -> ("data"=w462:string)  [unwired: 9 in]
        n160 = call "Select_Table_Vaule Enable_Disable.vi"("Action"=w472, "Table"=w457) -> ("Enable"=w471:bool)  [unwired: 8 in, 1 out]
        n161 = case shown="假" w471 {
          tunnel: w456 -> [w484 w512]
          tunnel: [w484 w512] -> w451
          tunnel: [w483 w503] -> w473
          tunnel: w472 -> [_ w509]
          tunnel: w457 -> [_ w513]
          tunnel: w455 -> [_ _]
          tunnel: [_ w492] -> w470
          tunnel: [_ w495] -> w459
          tunnel: w464 -> [_ w499]
          tunnel: w463 -> [_ w498]
          tunnel: w462 -> [_ w497]
          tunnel: w461 -> [_ w496]
          tunnel: [w482 w488] -> w452
          tunnel: [w482 w487] -> w445
          tunnel: [_ w485] -> _
          frame False {
            w483 = "Skip" ("software string")
            n162 = Initialize Array(w483, 5 ("维数大小")) -> (w482:string[])
          }
          frame True {
            w502 = string[] ["DDM_Pressure_corrected_after_Airwatts_Finetune", "DDM_Real_Power_after_Airwatts_Finetune", "Delta_V_after_Airwatts_Finetune", "Flow_rate_after_Airwatts_Finetune", "AW_after_Airwatts_Finetune"]
            n163 = Fract/Exp String To Number(string=w497) -> (number=w501:dbl)  [unwired: 3 in, 1 out]
            n164 = call "FCO_Read.vi"("VISA in"=w496) -> ("Pressure(Pa)"=w486:dbl)  [unwired: 7 in, 3 out]
            n165 = call "AW_Calculate_Tester_Parameter.vi"("Tester Parameter"=w498, "DDM Parameter"=w499, "AW_Box_Pressure/Stag Total-Static Pressure rise"=w486, "Orifice_Plate_Diameter"=w501) -> ("Calculate Tester Parameter"=w500:dbl[])  [unwired: 7 in]
            n166 = Number To Fractional String(number=w486) -> (F-format string=w485:string)  [unwired: 3 in]
            n167 = Number To Fractional String(number=w500) -> (F-format string=w488:string[])  [unwired: 3 in]
            n168 = Interleave 1D Arrays(w502, w488) -> (w506:string[])
            n169 = Build Array (concatenate)("" ("software string"), w488) -> (w508:string[])
            n170 = Array To Spreadsheet String(delimiter (Tab)=";" ("分隔符(Tab)"), array=w506, 3:"" ("格式字符串")) -> (spreadsheet string=w503:string)
            n171 = Build Array (concatenate)(w509, w502) -> (w510:string[])
            n172 = for {
              tunnel: w513 -> [w519]
              tunnel: w508 -> [w517] mode=indexing
              tunnel: w510 -> [w516] mode=indexing
              tunnel: [w515] -> w511 mode=indexing
              tunnel: [w514] -> w489 mode=indexing
              w524 = "UIdisplay" ("Process (\"\" - local)")
              n173 = call "Select_Table_Vaule.vi"("Vaule"=w517, "Action"=w516, "Table"=w519) -> ("Result"=w515:bool, "vaule"=w518:string[])  [unwired: 7 in]
              n174 = Append True/False String(1:w515, 2:"FAIL" ("真字符串"), 3:"PASS" ("真字符串")) -> (0:w514:string)  [unwired: 1 in]
              n175 = Build Array (concatenate)(w518, w517, w514) -> (w523:string[])
              n176 = Flatten To XML(anything=w523) -> (xml string=w522:string)
              n177 = call "AMC Send Local Message.vi"("Process (\"\" - local)"=w524, "Message Value"=w522, "Message Name"=w524) -> ()  [unwired: 7 in, 2 out]
            }
            n178 = Delete From Array(array=w511, length=1, index=0) -> (array with subset deleted=w495:bool[])  [unwired: 1 out]
            n179 = Build Array (concatenate)(w500, w486) -> (w492:dbl[])
            n180 = Delete From Array(array=w489, length=1, index=0) -> (array with subset deleted=w487:string[])  [unwired: 1 out]
          }
        }
        n181 = call <vilib>:"Space Constant.vi"() -> ("String"=w475:string)
        n182 = Concatenate Strings(w472, w475, w473) -> (w474:string)
        n183 = Index Array(array=w452) -> (element #1=w450:string, element #2=w449:string, element #3=w448:string, element #4=w447:string, element #5=w446:string)  [unwired: 5 in]
        n184 = Index Array(array=w445) -> (element #1=w444:string, element #2=w443:string, element #3=w442:string, element #4=w441:string, element #5=w440:string)  [unwired: 5 in]
        n185 = Unbundle By Name(w433) -> ("MES bool"=w438:refnum<vi>)
        n186 = Bundle By Name(cluster=w454, "daemon reference"=w451, "MAX.MAX finetune - Calculated Parameter - DDM Pressure Corrected"=w450, "MAX.MAX finetune - Calculated Parameter - DDM Real Power"=w449, "MAX.MAX finetune - Calculated Parameter - Delta V"=w448, "MAX.MAX finetune - Calculated Parameter - Flowrate"=w447, "MAX.MAX finetune - Calculated Parameter - Airwatt"=w446, "MAX_Status.MAX finetune - Calculated Parameter - DDM Pressure Corrected"=w444, "MAX_Status.MAX finetune - Calculated Parameter - DDM Real Power"=w443, "MAX_Status.MAX finetune - Calculated Parameter - Delta V"=w442, "MAX_Status.MAX finetune - Calculated Parameter - Flowrate"=w441, "MAX_Status.MAX finetune - Calculated Parameter - Airwatt"=w440) -> (w453:T1)
        n187 = call "HD_Config.vi"("Step"=enum16{"Initial", "Write", "Read"}."Read") -> ("HD Config out"=w439:T5)  [unwired: 9 in, 1 out]
        n188 = Unbundle By Name(w439) -> ("Fail_resume_mode"=w437:bool)
        n189 = property class="Bool (严格)"(reference=w438) -> ("Value"=w436:bool)  [unwired: 1 in, 2 out]
        n190 = Not(x=w436) -> (.not. x?=w435:bool)
        n191 = Or(x=w437, y=w435) -> (x .or. y?=w432:bool)
        n192 = Index Array(array=w459, index=4) -> (element=w430:bool)
        n193 = Bundle By Name(cluster=w469, "MAX.Cal_Tester_Parameter_after_Airwatts_Finetune"=w470, "MAX.Cal_Tester_Parameter_status_after_Airwatts_FineTune"=w459) -> (w476:T3)
        n194 = Select(t=TRUE, s=w432, f=w430) -> (s? t:f=w429:bool)
        n195 = call "LogStatus.vi"("error in (no error)"=w479, "last message"=w477, "message"=w474) -> ("error  out"=w478:errorcluster)  [unwired: 8 in]
        n196 = Select(t="Max_check_derate_status", s=w429, f="Airwatts_Finetune_Stop_motor") -> (s? t:f=w466:string)
      }
      frame "Airwatts_Finetune_Stop_motor" {
        n197 = Unbundle By Name(w528) -> ("Table"=w534:string[][], "daemon reference"=w538:refnum<k5>)
        n198 = call "Select_Table_Vaule Enable_Disable.vi"("Action"=w535, "Table"=w534) -> ("Enable"=w533:bool)  [unwired: 8 in, 1 out]
        n199 = case shown="真" w533 {
          tunnel: w538 -> [w545 w550]
          tunnel: [w545 w549] -> w525
          tunnel: ["" ("software string") w548] -> w529
          tunnel: w535 -> [_ w554]
          tunnel: w534 -> [_ w553]
          tunnel: [_ w546] -> w530
          frame False {
            (unwired) TRUE
          }
          frame True {
            w560 = "UIdisplay" ("Process (\"\" - local)")
            n200 = call "drive_motor.vi"("Power Mode"="STOP", "daemon reference in"=w550) -> ("error out"=w546:errorcluster, "response"=w548:string, "daemon reference out"=w549:refnum<k5>)  [unwired: 6 in, 1 out]
            n201 = call "Select_Table_Vaule.vi"("Vaule"=w548, "Action"=w554, "Table"=w553) -> ("Result"=w551:bool, "vaule"=w552:string[])  [unwired: 7 in]
            n202 = call "时间延迟"("error in (no error)"=w546) -> ()  [unwired: 10 in, 1 out]
            n203 = Append True/False String(1:w551, 2:"FAIL" ("真字符串"), 3:"PASS" ("真字符串")) -> (0:w555:string)  [unwired: 1 in]
            n204 = Build Array (concatenate)(w552, w548, w555) -> (w559:string[])
            n205 = Flatten To XML(anything=w559) -> (xml string=w558:string)
            n206 = call "AMC Send Local Message.vi"("Process (\"\" - local)"=w560, "Message Value"=w558, "Message Name"=w560) -> ()  [unwired: 7 in, 2 out]
          }
        }
        n207 = call <vilib>:"Space Constant.vi"() -> ("String"=w537:string)
        n208 = Concatenate Strings(w535, w537, w529) -> (w536:string)
        n209 = Bundle By Name(cluster=w528, "daemon reference"=w525) -> (w527:T1)
        n210 = case shown="无错误" w530 {
          tunnel: ["Finalization_NG_unit" "Error"] -> w532
          frame No Error {
          }
          frame Error {
          }
        }
        n211 = call "LogStatus.vi"("error in (no error)"=w530, "last message"=w539, "message"=w536) -> ("error  out"=w540:errorcluster)  [unwired: 8 in]
      }
    }
    n212 = call "6-AlarmStatus.vi"("Step"=enum16{"Initial", "Write", "Read"}."Read") -> ("AlarmValue Out"=w19:bool[])  [unwired: 9 in, 1 out]
    n213 = call "Stop.vi"("Step"=enum16{"Initial", "Write", "Read"}."Read") -> ("Stop Out"=w26:bool)  [unwired: 9 in, 1 out]
    n214 = call "Exit.vi"("Step"=enum16{"Initial", "Write", "Read"}."Read" ("step")) -> ("Exit Out"=w25:bool)  [unwired: 9 in, 1 out]
    n215 = Or Array Elements(Boolean array=w19) -> (logical OR=w18:bool)
    n216 = Compound Arithmetic op=OR(w24, w26, w25, w18) -> (w23:bool)
    n217 = call "AMC Run Step.vi"("Message Queue In"=w44, "Message Name"=w32, "Message Value"=w30, "error in (no error)"=w39, "Mli/Sig"=FALSE) -> ("Message Queue Out"=w43:T4, "error out"=w38:errorcluster)  [unwired: 13 in]
  }
  "Message Queue Out" <- w6
  "error out" <- w5
  "Data" <- w10
  "Flow" <- w7
  "Data out" <- w1
